vi "localise.vi"() -> ()   [LabVIEW 2016]
panel:
  out "stuff":cluster{dbl, dbl}[](graph)
  out "lidarPos":cluster{"xPos":dbl, "yPos":dbl, "theta":dbl}
  in  "landmarks":cluster{dbl, dbl}[](array[cluster])=[{0.0, 0.0}, {1045.0, 0.0}, {0.0, 4000.0}, {1045.0, 4000.0}, {6000.0, 0.0}, {6000.0, 4000.0}, {5035.0, 0.0}, {5035.0, 4000.0}]
  in  "point merge threshold":dbl=100.0
  out "rotated coordinate system":cluster{"Line":cluster{"X":dbl, "Y":dbl}[]}[](graph)=[{"Line"=[{"X"=4875.364468554468, "Y"=-181.33963012770346}, {"X"=4852.752184853944, "Y"=-189.0958192141975}, {"X"=4830.092735741714, "Y"=-196.71311592818483}, {"X"=4808.9364956042, "Y"=-208.94507233475179}, {"X"=4780.682915441052, "Y"=-199.14542201109134}, {"X"=4754.384597378405, "Y"=-194.86633064519674}, {"X"=4731.399241590487, "Y"=-200.92363554403482}, {"X"=4708.6695027964715, "Y"=-207.79610194101997}, {"X"=4684.775648004498, "Y"=-210.68966547950777}, {"X"=4661.986863653288, "Y"=-217.27587104156783}, {"X"=4639.158096096904, "Y"=-223.7221232680963}, {"X"=4619.181873799431, "Y"=-240.64129637134283}, {"X"=4596.72445242172, "Y"=-248.75730955534345}, {"X"=4573.703746936471, "Y"=-254.80252652544686}, {"X"=4550.156231819835, "Y"=-258.7673691163609}, {"X"=4528.509712831836, "Y"=-270.35259799092773}, {"X"=4496.497729685015, "Y"=-239.02618614387575}, {"X"=4473.538619990259, "Y"=-244.45660669015024}, {"X"=4453.201123871557, "Y"=-261.44876905485853}, {"X"=4430.1052468408925, "Y"=-266.613104523376}, {"X"=4406.978116816861, "Y"=-271.63562913740543}, {"X"=4402.516869914619, "Y"=-366.5963939235294}, {"X"=4378.776773303381, "Y"=-371.44775728191553}, {"X"=4016.6643720573857, "Y"=-184.5155449608328}, {"X"=3994.0487660964363, "Y"=-187.00278952130384}, {"X"=3971.217990913842, "Y"=-187.36127918351485}, {"X"=3948.585779371239, "Y"=-189.56961642142505}, {"X"=3925.5006968150883, "Y"=-186.65841872730198}, {"X"=3902.7918229304946, "Y"=-187.58960731348543}, {"X"=3880.159498496102, "Y"=-189.37808517945405}, {"X"=3857.09903168594, "Y"=-185.04220978622607}, {"X"=3833.975383762099, "Y"=-178.56650338054624}, {"X"=3811.8585360398097, "Y"=-187.9197334957098}, {"X"=3789.2258977826705, "Y"=-189.1502489880163}, {"X"=3766.4959424591943, "Y"=-188.243904779702}, {"X"=3743.862169062455, "Y"=-189.1960745279789}, {"X"=3721.354315175296, "Y"=-194.00719140993715}, {"X"=3698.6593279296276, "Y"=-193.6826253770737}, {"X"=3675.9934601757614, "Y"=-194.2184551012292}, {"X"=3653.324731311072, "Y"=-194.6151995885307}, {"X"=3630.6539948003874, "Y"=-194.8728439017732}, {"X"=3607.97562345001, "Y"=-191.99138534078702}, {"X"=3585.3377427102, "Y"=-187.97085376378345}, {"X"=3562.66860926447, "Y"=-191.81125834809563}, {"X"=3539.951796756734, "Y"=-195.51217198472432}, {"X"=3517.277690740343, "Y"=-195.07415616395292}, {"X"=3494.606699172145, "Y"=-194.4970228896659}, {"X"=3471.939675602154, "Y"=-193.78079389060622}, {"X"=3449.2774734309933, "Y"=-192.92549613238907}, {"X"=3426.6209458777726, "Y"=-191.9311618164934}, {"X"=3403.9709459479454, "Y"=-190.79782837904213}, {"X"=3381.2099975735023, "Y"=-191.52203499291227}, {"X"=3358.3022091020475, "Y"=-194.10153865253824}, {"X"=3335.4973580701767, "Y"=-194.54386256438193}, {"X"=3312.833042285723, "Y"=-192.8513561199734}, {"X"=3289.6776691762902, "Y"=-196.99878969308566}, {"X"=3266.9093951440886, "Y"=-196.02105634650388}, {"X"=3244.141439548919, "Y"=-194.90306841108986}, {"X"=3220.864802139731, "Y"=-198.61872889643155}, {"X"=3197.9614916352934, "Y"=-198.2110591192445}, {"X"=3175.277263429615, "Y"=-195.67457942933152}, {"X"=3152.007693840337, "Y"=-197.9626679594462}, {"X"=3129.3258548014196, "Y"=-195.14422574296668}, {"X"=3106.131977168781, "Y"=-196.1514276372368}, {"X"=3083.462115288954, "Y"=-193.05153141114988}, {"X"=3059.944141155934, "Y"=-195.7495409359385}, {"X"=3036.8256288278494, "Y"=-195.33200506461299}, {"X"=3013.535199662807, "Y"=-195.75743765272819}, {"X"=2989.730023886306, "Y"=-198.99602003762493}, {"X"=2964.5124034139135, "Y"=-209.96651124848268}, {"X"=2941.0609290320317, "Y"=-209.9357542620428}, {"X"=2904.379085672099, "Y"=-281.55213418374296}, {"X"=2789.552062093127, "Y"=-254.5246223646609}, {"X"=2766.529988551289, "Y"=-249.48112943853675}, {"X"=2741.532487512247, "Y"=-253.06988077801316}, {"X"=2718.520244051897, "Y"=-247.73177266645735}, {"X"=2695.5411878061436, "Y"=-242.2525645718888}, {"X"=2669.705574626602, "Y"=-248.2791094206391}, {"X"=2639.072200722142, "Y"=-272.54115478877384}, {"X"=2620.239607261427, "Y"=-250.12607425680517}, {"X"=2600.8696222588273, "Y"=-230.52040448444404}, {"X"=2574.293565720559, "Y"=-237.82052949011359}, {"X"=2551.3780387461265, "Y"=-231.45654971032445}, {"X"=2530.1606574432267, "Y"=-219.18590300588312}, {"X"=2508.4896445348645, "Y"=-208.7142170720531}, {"X"=2484.6010821776836, "Y"=-205.77728069575278}, {"X"=2461.8838573172898, "Y"=-198.86356138814972}, {"X"=2433.210564480137, "Y"=-210.88970641263268}, {"X"=2406.793414706115, "Y"=-215.08573855453687}, {"X"=2384.0205389293933, "Y"=-207.69442514542152}, {"X"=2361.2934440921063, "Y"=-200.16351913679637}, {"X"=2338.6129858565264, "Y"=-192.49330406301624}, {"X"=2315.980018129093, "Y"=-184.68406870334502}, {"X"=2293.395393028246, "Y"=-176.73610707107855}, {"X"=2264.0473517331984, "Y"=-187.45366365313384}, {"X"=2229.322955837718, "Y"=-212.0201293374671}, {"X"=2203.7550913262485, "Y"=-211.02750663514053}, {"X"=2181.0109385315222, "Y"=-202.39044988947717}, {"X"=2158.320209872944, "Y"=-193.61400023597616}, {"X"=2127.189617517972, "Y"=-206.0725272521504}, {"X"=2102.977286469537, "Y"=-200.67385690415676}, {"X"=2078.0144391875347, "Y"=-196.96685847714434}, {"X"=2044.5410314875958, "Y"=-213.38435894728354}, {"X"=2021.785414478626, "Y"=-203.77033872884704}, {"X"=1999.0892163567944, "Y"=-194.01687365053795}]}, {"Line"=[{"X"=995.1561569265573, "Y"=-120.2746516255329}, {"X"=990.8479691186076, "Y"=1267.3599305424295}, {"X"=977.1978637389684, "Y"=1283.4114152543848}, {"X"=963.646505377344, "Y"=1299.5463532737358}, {"X"=944.7929368001387, "Y"=1311.3117052596172}, {"X"=936.8420667751011, "Y"=1332.0641562303358}, {"X"=940.7364779704103, "Y"=1362.2297783899276}, {"X"=992.6762955394938, "Y"=1430.1922552666047}, {"X"=984.7473693279912, "Y"=1449.9310553634696}, {"X"=983.2886202921791, "Y"=1474.5858311674642}, {"X"=1038.4449660668279, "Y"=1542.2942488382926}, {"X"=1026.4809299503295, "Y"=1558.048508306483}, {"X"=1014.6137853722585, "Y"=1573.875881150741}, {"X"=976.2601861062503, "Y"=1570.223228197419}, {"X"=957.9951708726335, "Y"=1581.6581423355021}, {"X"=946.2741815106342, "Y"=1597.9052914528809}, {"X"=941.18381557668, "Y"=1618.8446376100087}, {"X"=1035.4542316465918, "Y"=1709.0536015780297}, {"X"=1037.6873121359445, "Y"=1733.9032615366507}, {"X"=1035.1673005512534, "Y"=1755.2830533755748}, {"X"=1032.8128759176288, "Y"=1776.627065912406}, {"X"=1034.7918620045143, "Y"=1800.6953749366378}, {"X"=1024.4134141596182, "Y"=1816.4671851017908}, {"X"=1015.8127079164447, "Y"=1833.3863556799192}, {"X"=1025.8839062712937, "Y"=1862.1577194348454}, {"X"=1020.9645951345497, "Y"=1881.1728379933504}, {"X"=1006.82910819158, "Y"=1894.3958377366096}, {"X"=1030.3100502453976, "Y"=1930.6642927244054}, {"X"=1030.1519372868106, "Y"=1952.136655072785}, {"X"=1029.3004603365107, "Y"=1973.040970826681}, {"X"=1034.6486208208826, "Y"=1997.4350924689477}, {"X"=1036.7349309586402, "Y"=2019.7053719504383}, {"X"=1052.0328316602431, "Y"=2049.314882869931}, {"X"=1044.923639308267, "Y"=2065.955094484733}, {"X"=1052.7981056635122, "Y"=2090.857172076369}, {"X"=1044.1997181730085, "Y"=2106.513035793635}, {"X"=1035.697555118571, "Y"=2122.2213635075027}, {"X"=1027.2919366018336, "Y"=2137.9815638083105}, {"X"=973.7644027699575, "Y"=2130.2078304203374}, {"X"=1038.1094935815977, "Y"=2647.5230014110284}, {"X"=1052.8931430954117, "Y"=2669.7665030188023}, {"X"=1057.3733887850622, "Y"=2688.4515319824445}, {"X"=1052.4416852255154, "Y"=2704.0680727452964}, {"X"=1047.6058957966343, "Y"=2719.714579895345}, {"X"=1053.4051578916715, "Y"=2738.5417213351366}, {"X"=1051.6603564800585, "Y"=2755.023449184703}, {"X"=1050.021828763001, "Y"=2771.4978886682547}, {"X"=1046.5630241118151, "Y"=2787.4267685584864}, {"X"=1045.133311119083, "Y"=2803.8964142840096}, {"X"=1046.7087363121373, "Y"=2821.12760935855}, {"X"=1054.2071036963334, "Y"=2839.819320844825}, {"X"=1053.1127473126949, "Y"=2856.1876654653834}, {"X"=1056.978250286315, "Y"=2873.7401653601373}, {"X"=1053.1834638463438, "Y"=2889.3556426410773}, {"X"=1061.1707740855086, "Y"=2907.720368708814}, {"X"=1058.5596338716723, "Y"=2923.5306899638895}, {"X"=1080.4610293828596, "Y"=2944.731258270807}, {"X"=1079.05712939688, "Y"=2960.6197601364106}, {"X"=1075.7950105001619, "Y"=2976.0981284781265}, {"X"=1075.5690111418248, "Y"=2992.187847238236}, {"X"=1072.5006560489983, "Y"=3007.6870240108883}, {"X"=1057.7349664870621, "Y"=3020.982777577399}, {"X"=1016.4744379708436, "Y"=3029.6047721947734}, {"X"=985.074506559165, "Y"=3040.446234099636}, {"X"=961.5990224884686, "Y"=3052.991854810011}, {"X"=958.9058992251366, "Y"=3069.189193668247}, {"X"=932.602007282233, "Y"=3081.6843913440134}, {"X"=1024.2156184414202, "Y"=3176.6568081451514}, {"X"=1032.2096938775303, "Y"=3193.652250239258}, {"X"=1030.378317349322, "Y"=3209.413682270658}, {"X"=1028.6436856251103, "Y"=3225.1860547126794}, {"X"=1024.0209520220938, "Y"=3240.668273481939}, {"X"=1022.4782145399163, "Y"=3256.479065625435}]}, {"Line"=[{"X"=-27.88704701562665, "Y"=3179.6883172654543}, {"X"=-29.784148604247548, "Y"=3201.9546434830118}, {"X"=-40.51875378113118, "Y"=3223.5507218893886}, {"X"=-42.14648292623542, "Y"=3245.8937291052093}, {"X"=-43.63708731480574, "Y"=3268.2463032785063}, {"X"=-42.9938027953026, "Y"=3290.7223069817924}, {"X"=-44.20932825047976, "Y"=3313.079236326757}, {"X"=-45.287651284163985, "Y"=3335.4432031328274}, {"X"=-45.22949075787301, "Y"=3357.852331327238}, {"X"=-44.03415040060372, "Y"=3380.287382811384}, {"X"=-44.70009529764866, "Y"=3402.64900957201}, {"X"=-45.22881929609821, "Y"=3425.0143015424014}, {"X"=-45.620302489793175, "Y"=3447.3824166819586}, {"X"=-45.874530139612034, "Y"=3469.7525128437887}, {"X"=-45.99149267402754, "Y"=3492.1237478064127}, {"X"=-45.97118568946689, "Y"=3514.49527930548}, {"X"=-44.81366107226677, "Y"=3536.8561536378656}, {"X"=-45.518771389693484, "Y"=3559.235862831427}, {"X"=-44.086931606495455, "Y"=3581.580848823444}, {"X"=-43.51776202187057, "Y"=3603.939010150847}, {"X"=-42.81141605282983, "Y"=3626.293258233267}, {"X"=-42.967088446615435, "Y"=3648.6835313502697}, {"X"=-45.98180211856061, "Y"=3671.2211979291474}, {"X"=-48.856943965644405, "Y"=3693.801451165101}, {"X"=-47.59911191565743, "Y"=3716.1867682169914}, {"X"=-46.20394982073867, "Y"=3738.563945959246}, {"X"=-44.67151020795109, "Y"=3760.9321419037724}, {"X"=-51.97476173527639, "Y"=3783.988273787092}, {"X"=-52.15648631405884, "Y"=3806.558313333936}, {"X"=-50.206729051451475, "Y"=3828.9617533810065}, {"X"=-46.12875527743017, "Y"=3851.161074065816}, {"X"=-43.90543409027123, "Y"=3873.5266890161834}]}, {"Line"=[{"X"=-57.451206048306176, "Y"=3897.6074387832673}, {"X"=1335.6105985632566, "Y"=3873.584848007716}, {"X"=1337.9454985878674, "Y"=3887.471847546513}, {"X"=1353.1652358742085, "Y"=3899.0708492433396}, {"X"=1355.6561846014824, "Y"=3912.8496557857657}, {"X"=1820.0951553792638, "Y"=3850.049630903437}, {"X"=1822.2765257416634, "Y"=3860.964332131124}, {"X"=1949.8064262901478, "Y"=3845.6257647900497}, {"X"=2047.7518614123712, "Y"=3835.0667340265845}, {"X"=2074.2413420170706, "Y"=3839.160017676214}, {"X"=2132.890864786777, "Y"=3835.582754881576}, {"X"=2166.127558146054, "Y"=3837.251865067938}, {"X"=2200.3003394848, "Y"=3838.2910881971834}, {"X"=2248.018436192918, "Y"=3835.5515625440557}, {"X"=2277.236404755542, "Y"=3836.9294749587143}, {"X"=2307.3868846214937, "Y"=3837.7089485806855}, {"X"=2344.25776130767, "Y"=3836.3204275151534}, {"X"=2371.41812317585, "Y"=3837.1388021857606}, {"X"=2396.6148897993025, "Y"=3838.177877081358}, {"X"=2414.0890428141442, "Y"=3841.132234810093}, {"X"=2450.739877896451, "Y"=3838.2383357080275}, {"X"=2474.8609031479305, "Y"=3838.6547101915307}, {"X"=2494.1640463756876, "Y"=3840.2584953705154}, {"X"=2511.535949867143, "Y"=3842.238238027806}, {"X"=2537.4588200341204, "Y"=3841.26564561455}, {"X"=2560.4772677834208, "Y"=3840.9229960049315}, {"X"=2579.6576251688384, "Y"=3841.5807929669136}, {"X"=2592.1821197265217, "Y"=3844.2791312308555}, {"X"=2624.5313575165155, "Y"=3839.926356041171}, {"X"=2642.654053105019, "Y"=3840.2127833632244}, {"X"=2653.221356629601, "Y"=3843.014869149585}, {"X"=2670.353311050435, "Y"=3843.2754487654347}, {"X"=2686.5163060590426, "Y"=3843.6910544427697}, {"X"=2712.9203209596462, "Y"=3839.9847688259915}, {"X"=2718.749345719235, "Y"=3843.9669814527606}, {"X"=2735.745373534478, "Y"=3843.4587902979656}, {"X"=2759.190584115213, "Y"=3840.130160614261}, {"X"=2762.2181156127335, "Y"=3844.902180614331}, {"X"=2778.185428757569, "Y"=3844.2409192609425}, {"X"=2791.3526756724646, "Y"=3844.5729311160676}, {"X"=2798.98739923077, "Y"=3847.1423532341078}, {"X"=2804.792835674701, "Y"=3850.437677491615}, {"X"=2817.9091475083846, "Y"=3850.4039075822907}, {"X"=2837.3651516827986, "Y"=3847.321303884745}, {"X"=2852.215704506808, "Y"=3846.113633672166}, {"X"=2861.5927811261063, "Y"=3847.2906262986685}, {"X"=2874.5650046463807, "Y"=3846.6411220791524}, {"X"=2883.9025697924535, "Y"=3847.5923912431745}, {"X"=2896.8119198019726, "Y"=3846.6735119206733}, {"X"=2900.740692773926, "Y"=3850.0863054415463}, {"X"=2910.9248129571906, "Y"=3850.291859171631}, {"X"=2923.750724150955, "Y"=3849.0099094777147}, {"X"=2930.33394718425, "Y"=3850.832406864265}, {"X"=2937.7968458711803, "Y"=3852.1178533699235}, {"X"=2955.810589401053, "Y"=3847.6262407704303}, {"X"=2966.7268074487856, "Y"=3846.769467508303}, {"X"=2977.607927778653, "Y"=3845.7920016946864}, {"X"=2984.9682824182264, "Y"=3846.658313571755}, {"X"=2988.8431566734257, "Y"=3849.432844556857}, {"X"=3000.514385824566, "Y"=3847.6578754993225}, {"X"=3004.3827878484135, "Y"=3850.315766971416}, {"X"=3013.414194881955, "Y"=3849.8658217574493}, {"X"=3017.2833293798044, "Y"=3852.4234410213294}, {"X"=3034.8014845147404, "Y"=3846.582801208108}, {"X"=3037.787979177994, "Y"=3849.5162995387154}, {"X"=3053.4792714726036, "Y"=3844.4286476033662}, {"X"=3057.2883738551773, "Y"=3846.698847484733}, {"X"=3063.622898309917, "Y"=3847.304772185103}, {"X"=3067.436117579296, "Y"=3849.492075934472}, {"X"=3070.4232538474694, "Y"=3852.199474636885}, {"X"=3088.3501096376754, "Y"=3844.823708135362}, {"X"=3090.4755397996805, "Y"=3847.956641634519}, {"X"=3092.620153269628, "Y"=3851.0764747627854}, {"X"=3108.7039247689136, "Y"=3844.4243987619507}, {"X"=3110.8265216598475, "Y"=3847.432451116179}, {"X"=3113.779256429665, "Y"=3849.8433771302675}, {"X"=3119.167495430773, "Y"=3850.46412448307}, {"X"=3125.3494169762807, "Y"=3850.4380459300096}, {"X"=3131.5127639763296, "Y"=3850.3494108499426}, {"X"=3136.859859086742, "Y"=3850.8022375567853}, {"X"=3141.401329549159, "Y"=3851.811397570802}, {"X"=3149.8860258047935, "Y"=3849.7104662920415}, {"X"=3156.755647605926, "Y"=3848.755564931598}, {"X"=3160.4680859852774, "Y"=3850.2223530309775}, {"X"=3169.629505439559, "Y"=3847.2610508130756}, {"X"=3172.5427398878355, "Y"=3849.262495520778}, {"X"=3178.5462320761003, "Y"=3848.691441682683}, {"X"=3183.7599215441505, "Y"=3848.7021610014317}, {"X"=3186.6699549419614, "Y"=3850.602729385154}, {"X"=3191.1048479470255, "Y"=3851.1776681789074}, {"X"=3199.3041794662954, "Y"=3848.4305661201684}, {"X"=3205.953045974128, "Y"=3846.91785486327}, {"X"=3208.0891117368533, "Y"=3849.3291508889447}, {"X"=3211.7247329793054, "Y"=3850.3873813652654}, {"X"=3220.5264570839636, "Y"=3846.6927028749683}, {"X"=3224.129112653411, "Y"=3847.656548975117}, {"X"=3226.2693687986784, "Y"=3849.9563048465648}, {"X"=3229.875165629684, "Y"=3850.866936291162}, {"X"=3232.7565121495086, "Y"=3852.4389601497064}, {"X"=3239.9466149416203, "Y"=3849.8078900025016}, {"X"=3245.66451699703, "Y"=3848.504469820765}, {"X"=3249.935468453753, "Y"=3848.5553381506397}, {"X"=3254.193623585364, "Y"=3848.566995039661}, {"X"=3257.0388209403313, "Y"=3849.9680409094553}, {"X"=3266.843418073042, "Y"=3844.1623046162176}, {"X"=3268.961429853259, "Y"=3846.2000362149047}, {"X"=3273.1518722403007, "Y"=3846.0437853508993}, {"X"=3275.281309814408, "Y"=3848.0427735841577}, {"X"=3278.1006556937873, "Y"=3849.2933038797487}, {"X"=3283.6157288974155, "Y"=3847.564372453343}, {"X"=3287.091515385653, "Y"=3848.0118967166973}, {"X"=3293.2169619535393, "Y"=3845.43909386024}, {"X"=3297.98004039561, "Y"=3844.307920327957}, {"X"=3298.1339382930623, "Y"=3848.4219866620697}, {"X"=3302.227969769491, "Y"=3847.9882440721253}, {"X"=3304.368790968698, "Y"=3849.8087881210113}, {"X"=3309.0838801357822, "Y"=3848.5452785552375}, {"X"=3315.044360347663, "Y"=3845.6939158132923}, {"X"=3317.1708625483957, "Y"=3847.4358631580535}, {"X"=3319.9345577199, "Y"=3848.3853441814854}, {"X"=3322.077482158057, "Y"=3850.09723517388}, {"X"=3324.2308702219293, "Y"=3851.7959452032464}, {"X"=3327.006733363762, "Y"=3852.6906241612837}, {"X"=3334.033772019595, "Y"=3848.002824088936}, {"X"=3337.3787684930608, "Y"=3848.03173527967}, {"X"=3339.5191948454476, "Y"=3849.6365972635535}, {"X"=3341.6694281529244, "Y"=3851.2282956271647}, {"X"=3346.767123842757, "Y"=3848.7608212416217}, {"X"=3348.9118470493695, "Y"=3850.3080636351965}, {"X"=3352.7987426764153, "Y"=3849.393100071594}, {"X"=3354.9472319294746, "Y"=3850.9033212452873}, {"X"=3358.239970891585, "Y"=3850.7536005880743}, {"X"=3360.959154637208, "Y"=3851.403577455099}, {"X"=3363.677191444651, "Y"=3852.0334219310885}, {"X"=3365.2894164277122, "Y"=3854.310516297719}, {"X"=3371.844919137942, "Y"=3849.0476458548715}, {"X"=3373.9909301848866, "Y"=3850.4410083898674}, {"X"=3376.145450345569, "Y"=3851.821177018968}, {"X"=3379.371667575448, "Y"=3851.4941520588377}, {"X"=3384.69111397845, "Y"=3847.7399654916867}, {"X"=3386.828859423541, "Y"=3849.054529873674}, {"X"=3390.0065395382076, "Y"=3848.6427205080895}, {"X"=3392.6604127610813, "Y"=3849.064887325544}, {"X"=3394.300734152325, "Y"=3851.193411142247}, {"X"=3398.459886789198, "Y"=3848.9850752782663}, {"X"=3401.5945661769583, "Y"=3848.4770922592916}, {"X"=3402.7576461014837, "Y"=3851.4320045593067}, {"X"=3405.885855720585, "Y"=3850.8855924523987}, {"X"=3410.4359883800344, "Y"=3847.6801482663996}, {"X"=3412.5728821535454, "Y"=3848.836746194794}, {"X"=3413.781058878635, "Y"=3851.7477874381552}, {"X"=3416.8677585572095, "Y"=3851.1104984818016}, {"X"=3419.0255794876925, "Y"=3852.227567234926}, {"X"=3422.5448335937085, "Y"=3850.6546219796846}, {"X"=3424.699750449227, "Y"=3851.7368654369866}, {"X"=3426.8612672600616, "Y"=3852.805866200107}, {"X"=3429.8993825310763, "Y"=3852.060761711229}, {"X"=3432.921802718256, "Y"=3851.2917249140414}, {"X"=3437.200222193895, "Y"=3847.781874666123}, {"X"=3439.337236319723, "Y"=3848.7742484281425}, {"X"=3442.3059227489016, "Y"=3847.9318582710193}, {"X"=3444.8509763286847, "Y"=3847.979569017834}, {"X"=3446.5874559424906, "Y"=3849.8408085484066}, {"X"=3448.736926737098, "Y"=3850.7755445681214}, {"X"=3450.8920925009197, "Y"=3851.6970740868423}, {"X"=3451.129480366653, "Y"=3857.220615844183}, {"X"=3453.324147305234, "Y"=3858.1273436031706}, {"X"=3456.6443028904364, "Y"=3856.237482736209}, {"X"=3459.935702110019, "Y"=3854.320465760287}, {"X"=3462.1124082875845, "Y"=3855.173214152968}, {"X"=3466.787586324898, "Y"=3849.471676739122}, {"X"=3469.2848546564674, "Y"=3849.3458898825334}, {"X"=3471.4308614151137, "Y"=3850.1413665986074}, {"X"=3473.920631762058, "Y"=3849.982846586403}, {"X"=3476.7367473982727, "Y"=3848.8641147467633}, {"X"=3478.8796577604844, "Y"=3849.6138765778364}, {"X"=3481.670224839258, "Y"=3848.4566892892262}, {"X"=3483.81054241454, "Y"=3849.1761875414713}, {"X"=3485.3354259488456, "Y"=3851.784075048413}, {"X"=3487.192026363989, "Y"=3853.4336728215594}, {"X"=3489.362778189773, "Y"=3854.1191962462844}, {"X"=3491.537695444426, "Y"=3854.79138728342}, {"X"=3493.716696243542, "Y"=3855.4502206253537}, {"X"=3497.0220737667746, "Y"=3852.2563650364664}, {"X"=3500.009514130937, "Y"=3849.9970038952742}, {"X"=3502.6965259216036, "Y"=3848.677550083562}, {"X"=3504.837802859068, "Y"=3849.2680292201253}, {"X"=3506.9826625994683, "Y"=3849.8453586127957}, {"X"=3508.6289858507666, "Y"=3852.345480705146}, {"X"=3510.7926571105445, "Y"=3852.8994899041413}, {"X"=3512.9596869763614, "Y"=3853.4402126368004}, {"X"=3515.1299938607685, "Y"=3853.96762854522}, {"X"=3517.3034960529376, "Y"=3854.481717772487}, {"X"=3520.1437371745833, "Y"=3852.05678134011}, {"X"=3522.7358611314803, "Y"=3850.5870118029275}, {"X"=3525.5161499645315, "Y"=3848.120892914938}, {"X"=3527.4503614688483, "Y"=3849.550496994353}, {"X"=3529.596528723903, "Y"=3849.9890730183956}, {"X"=3531.7453466298593, "Y"=3850.4144721516536}, {"X"=3533.896734284937, "Y"=3850.82667837809}, {"X"=3536.050610690607, "Y"=3851.2256761783733}, {"X"=3538.2068947546404, "Y"=3851.6114505304627}, {"X"=3540.6995920992354, "Y"=3850.012087823839}, {"X"=3543.0093327946784, "Y"=3849.3824034657328}, {"X"=3545.154175753993, "Y"=3849.7255146007737}, {"X"=3547.301083627591, "Y"=3850.0554587678553}, {"X"=3549.449975585606, "Y"=3850.3722235447667}, {"X"=3551.737491710125, "Y"=3849.6851874094323}, {"X"=3553.8840282116666, "Y"=3849.9747378683464}, {"X"=3556.156855341715, "Y"=3849.258899194384}, {"X"=3558.1822290543146, "Y"=3850.5142993276227}, {"X"=3560.446100602967, "Y"=3849.7706234698526}, {"X"=3562.5929973932184, "Y"=3850.006737300836}, {"X"=3564.7413025359765, "Y"=3850.229673575984}, {"X"=3566.890935148765, "Y"=3850.439423901873}, {"X"=3569.0418142991325, "Y"=3850.635980381521}, {"X"=3571.0301877520556, "Y"=3852.8126272943173}, {"X"=3573.195550684427, "Y"=3852.9837411225744}, {"X"=3575.361922789166, "Y"=3853.141565312486}, {"X"=3577.529222503586, "Y"=3853.28609392206}, {"X"=3579.6973682300777, "Y"=3853.417321509876}, {"X"=3581.866278339181, "Y"=3853.535243135289}, {"X"=3584.035871172656, "Y"=3853.639854358617}, {"X"=3586.206065046558, "Y"=3853.7311512413066}, {"X"=3588.376778254314, "Y"=3853.8091303460815}, {"X"=3590.5479290698, "Y"=3853.8737887370726}, {"X"=3592.7194357504145, "Y"=3853.9251239799287}, {"X"=3594.862353356768, "Y"=3855.962925860221}, {"X"=3597.0383014495974, "Y"=3856.9877145528917}, {"X"=3599.2287926403974, "Y"=3856.9991670007207}, {"X"=3601.4193128667184, "Y"=3856.997178631689}, {"X"=3603.650225367152, "Y"=3860.9815450334945}, {"X"=3605.735123307596, "Y"=3852.953408200922}, {"X"=3607.900696744767, "Y"=3852.911573897694}, {"X"=3610.00894171823, "Y"=3850.8572659724764}, {"X"=3612.3001664397284, "Y"=3854.7868457335403}, {"X"=3614.3545263399055, "Y"=3851.707190107846}, {"X"=3616.5592007860246, "Y"=3852.611390725439}, {"X"=3618.7224718832185, "Y"=3852.5031475697515}, {"X"=3620.885038089928, "Y"=3852.381632869794}, {"X"=3623.046817986758, "Y"=3852.2468512005257}, {"X"=3625.2077301839167, "Y"=3852.0988076364006}, {"X"=3627.290164448009, "Y"=3850.940517644231}, {"X"=3629.2756915871423, "Y"=3848.7734707257623}, {"X"=3631.594689547098, "Y"=3850.579200170835}, {"X"=3633.265872973202, "Y"=3845.401768517955}, {"X"=3635.3845921617844, "Y"=3845.1911508679564}, {"X"=3637.7181288761512, "Y"=3846.955822481886}, {"X"=3640.0746453054317, "Y"=3848.704778865509}, {"X"=3642.2135032112865, "Y"=3848.452321195642}, {"X"=3644.3507718026044, "Y"=3848.186744492827}, {"X"=3646.8836900193755, "Y"=3850.8816319076377}, {"X"=3649.451334095426, "Y"=3853.558433015227}, {"X"=3651.1860171434532, "Y"=3850.2798761690287}, {"X"=3653.334330496239, "Y"=3849.9592107525073}, {"X"=3655.4806358416267, "Y"=3849.625369569499}, {"X"=3657.4620703035835, "Y"=3848.2917031403795}, {"X"=3659.260400212996, "Y"=3845.961276686561}, {"X"=3661.3820631395324, "Y"=3845.5911490833273}, {"X"=3663.863246490962, "Y"=3847.175007377597}, {"X"=3666.7400578446986, "Y"=3850.7060944421787}, {"X"=3668.8906936232233, "Y"=3850.289983202648}, {"X"=3671.0387357060704, "Y"=3849.860683743234}, {"X"=3673.1841032206685, "Y"=3849.4182122268194}, {"X"=3675.537714597933, "Y"=3849.9400715455736}, {"X"=3677.683484534923, "Y"=3849.469993319187}, {"X"=3679.8263297326275, "Y"=3848.9867577450727}, {"X"=3681.9661695141353, "Y"=3848.4903830167773}, {"X"=3684.572772049296, "Y"=3849.9249151288}, {"X"=3686.95916301393, "Y"=3850.3699530038452}, {"X"=3688.8605208682325, "Y"=3848.8607284161208}, {"X"=3691.2521934413376, "Y"=3849.2764480925457}, {"X"=3693.3935956407463, "Y"=3848.7099601291775}, {"X"=3696.3253720530747, "Y"=3851.0233933783284}, {"X"=3698.4773978060916, "Y"=3850.425744090443}, {"X"=3700.6257159407405, "Y"=3849.8149014713545}, {"X"=3702.2055738950803, "Y"=3847.272257263343}, {"X"=3703.758038867192, "Y"=3844.7234679716976}, {"X"=3705.8712690867633, "Y"=3844.0803312919206}, {"X"=3708.5804050535194, "Y"=3845.332152627602}]}]
  out "angle deviation":dbl=-12.54564800056658 format="%0.2f"
  in  "max angle deviation":dbl=30.0
  out "split&merge":cluster{"Line":cluster{"X":dbl, "Y":dbl}[]}[](graph)=[{"Line"=[{"X"=4045.262015510834, "Y"=-370.47254705975547}, {"X"=4021.5048604927456, "Y"=-373.1317628736815}, {"X"=3997.731836054895, "Y"=-375.64515746583857}, {"X"=3974.4237446268694, "Y"=-382.9895518092235}, {"X"=3948.973422153729, "Y"=-367.28671688954455}, {"X"=3924.2325152064327, "Y"=-357.3973448535103}, {"X"=3900.4802229985116, "Y"=-358.3172025621179}, {"X"=3876.8003772484603, "Y"=-360.08828281881506}, {"X"=3852.848497603733, "Y"=-357.72259724044125}, {"X"=3829.173196937117, "Y"=-359.2014259177531}, {"X"=3805.4892680291655, "Y"=-360.5349578426094}, {"X"=3782.314874586134, "Y"=-372.7109737888577}, {"X"=3758.6307242397825, "Y"=-375.7550610593494}, {"X"=3734.846552078191, "Y"=-376.65544089136483}, {"X"=3711.0000422297094, "Y"=-375.4106867047012}, {"X"=3687.3538586650116, "Y"=-382.0172981809769}, {"X"=3662.9108581038413, "Y"=-344.48530026226535}, {"X"=3639.320355486937, "Y"=-344.7989426814479}, {"X"=3615.7774597291873, "Y"=-356.96773019486045}, {"X"=3592.111253634981, "Y"=-356.9919325402784}, {"X"=3568.4453445476156, "Y"=-356.8709213194161}, {"X"=3543.4634903042615, "Y"=-448.5952721279782}, {"X"=3519.2364294721056, "Y"=-448.174039435899}, {"X"=3206.375015694224, "Y"=-187.04805660711145}, {"X"=3183.7591240020847, "Y"=-184.5634114706845}, {"X"=3161.3956031641924, "Y"=-179.95410067521016}, {"X"=3138.8240858920867, "Y"=-177.1936005936277}, {"X"=3116.9225625935896, "Y"=-169.33743194447243}, {"X"=3094.5536322950015, "Y"=-165.31362496769452}, {"X"=3072.0732055742583, "Y"=-162.14326586595462}, {"X"=3050.50517501786, "Y"=-152.90178314690638}, {"X"=3029.3402803672284, "Y"=-141.5578375729042}, {"X"=3005.7198268817183, "Y"=-145.8835795782761}, {"X"=2983.360292949494, "Y"=-142.16851225868822}, {"X"=2961.369928605174, "Y"=-136.34646752894514}, {"X"=2939.069748166673, "Y"=-132.35945388277014}, {"X"=2916.0542503508345, "Y"=-132.16660019014535}, {"X"=2893.971646836575, "Y"=-126.92003834235948}, {"X"=2871.7305746338234, "Y"=-122.51965406356612}, {"X"=2849.516921363317, "Y"=-117.98288396725366}, {"X"=2827.3315233565468, "Y"=-113.3098988602519}, {"X"=2805.820540469126, "Y"=-105.57110400824695}, {"X"=2784.596507850818, "Y"=-96.72922875644326}, {"X"=2761.6344368770942, "Y"=-95.5538074919159}, {"X"=2738.656125118518, "Y"=-94.23186914869939}, {"X"=2716.6185475221346, "Y"=-88.87910208996846}, {"X"=2694.614228738148, "Y"=-83.39121576148591}, {"X"=2672.6439972167227, "Y"=-77.76841677907123}, {"X"=2650.708680124659, "Y"=-72.01091683792765}, {"X"=2628.809103314247, "Y"=-66.11893270467408}, {"X"=2606.946091292176, "Y"=-60.092686209182375}, {"X"=2584.5712899521213, "Y"=-55.85552783159346}, {"X"=2561.650151837172, "Y"=-53.3974718317445}, {"X"=2539.293725910705, "Y"=-48.87562477295114}, {"X"=2517.538201938755, "Y"=-42.30044684778477}, {"X"=2494.034809091436, "Y"=-41.3191040202214}, {"X"=2472.0225479250194, "Y"=-35.41905120318597}, {"X"=2450.0410633250167, "Y"=-29.382161789984366}, {"X"=2426.5130901879893, "Y"=-27.95301449719682}, {"X"=2404.2451890722396, "Y"=-22.58008172179325}, {"X"=2382.6535537697796, "Y"=-15.176756558716079}, {"X"=2359.4425731187703, "Y"=-12.355658331004179}, {"X"=2337.9145170954243, "Y"=-4.677621956337134}, {"X"=2315.0556519473794, "Y"=-0.6226620999336774}, {"X"=2293.6004238067435, "Y"=7.327506432634436}, {"X"=2270.057927743648, "Y"=9.802429024614412}, {"X"=2247.5821062096375, "Y"=15.231737897677704}, {"X"=2224.75536526262, "Y"=19.875548974426238}, {"X"=2200.815103181707, "Y"=21.88519100999474}, {"X"=2173.8166160981887, "Y"=16.65434452990621}, {"X"=2150.9317674680565, "Y"=21.778434678614303}, {"X"=2099.569445467065, "Y"=-40.16004596176299}, {"X"=1993.354962067471, "Y"=11.164560761459143}, {"X"=1971.9781148912214, "Y"=21.088425727543836}, {"X"=1946.7979336116412, "Y"=23.015253457493145}, {"X"=1925.494677341689, "Y"=33.224563893850245}, {"X"=1904.2544652507022, "Y"=43.564396465946174}, {"X"=1877.726652128255, "Y"=43.29368976613068}, {"X"=1842.55456574985, "Y"=26.26504384210375}, {"X"=1829.0405780564897, "Y"=52.23569166488596}, {"X"=1814.3917771697875, "Y"=75.5807390798177}, {"X"=1786.8645563340388, "Y"=74.22769832520271}, {"X"=1765.8785444190275, "Y"=85.41737745628188}, {"X"=1747.8331626322108, "Y"=102.00382481748511}, {"X"=1728.9542149611082, "Y"=116.9328013933573}, {"X"=1706.27398723018, "Y"=124.98862393636955}, {"X"=1685.60095559409, "Y"=136.67184194320134}, {"X"=1655.000000000001, "Y"=131.16117927853338}, {"X"=1628.3021546343343, "Y"=132.80359845458497}, {"X"=1607.6785425781395, "Y"=144.9650955174202}, {"X"=1587.1299402987506, "Y"=157.25290774813675}, {"X"=1566.6571214394316, "Y"=169.66657251754714}, {"X"=1546.2608567902394, "Y"=182.2056224581911}, {"X"=1525.9419142590123, "Y"=194.86958548192388}, {"X"=1494.9665691389255, "Y"=190.7828335152658}, {"X"=1455.735015665709, "Y"=174.34567686930814}, {"X"=1430.993243345882, "Y"=180.86838320792322}, {"X"=1410.668265549114, "Y"=194.23964018468632}, {"X"=1390.425714854734, "Y"=207.7353571705712}, {"X"=1357.3322111709276, "Y"=202.3364045208432}, {"X"=1334.8706766640394, "Y"=212.86551103190004}, {"X"=1311.3090852839077, "Y"=221.9063623965808}, {"X"=1275.0687472590512, "Y"=213.15186386282812}, {"X"=1254.9447924102292, "Y"=227.47924783415692}, {"X"=1234.9091275645433, "Y"=241.92984036216785}]}, {"Line"=[{"X"=270.96481001367874, "Y"=531.983035117094}, {"X"=568.1778192565093, "Y"=1887.4212377834735}, {"X"=558.3402951796288, "Y"=1906.0545053007447}, {"X"=548.617287871481, "Y"=1924.7477839649912}, {"X"=532.7695198753122, "Y"=1940.3275402206798}, {"X"=529.5162834990319, "Y"=1962.3115573360112}, {"X"=539.8702058904678, "Y"=1990.9109889727677}, {"X"=605.3325001870285, "Y"=2045.968512870534}, {"X"=601.8805011027116, "Y"=2066.9583152148466}, {"X"=605.8120277476805, "Y"=2091.3412809272986}, {"X"=674.3588639641607, "Y"=2145.452125934663}, {"X"=666.1025888247354, "Y"=2163.429021451132}, {"X"=657.9567732645942, "Y"=2181.4562381095116}, {"X"=619.7255133273352, "Y"=2186.221866490394}, {"X"=604.3804690989409, "Y"=2201.3512306693083}, {"X"=596.4685017416655, "Y"=2219.7564532597535}, {"X"=596.0480668191567, "Y"=2241.301551943805}, {"X"=707.6625662145384, "Y"=2308.879448114789}, {"X"=715.2401057472161, "Y"=2332.650715290977}, {"X"=717.4243259383866, "Y"=2354.0674176426273}, {"X"=719.7624075179106, "Y"=2375.413226623674}, {"X"=726.9221966011937, "Y"=2398.476992697342}, {"X"=720.2174633677091, "Y"=2416.1266025463633}, {"X"=715.4972516675775, "Y"=2434.5100212284015}, {"X"=731.5776225251552, "Y"=2460.4067793595614}, {"X"=730.9061825143826, "Y"=2480.0364386578276}, {"X"=719.9804701443845, "Y"=2496.014189517481}, {"X"=750.778902136793, "Y"=2526.316203538756}, {"X"=755.2887344326768, "Y"=2547.3102207148654}, {"X"=758.99836842379, "Y"=2567.9003650996783}, {"X"=769.5176591565032, "Y"=2590.550321252946}, {"X"=776.3916464972967, "Y"=2611.8356762232834}, {"X"=797.7559831999147, "Y"=2637.415238768894}, {"X"=794.4310781670474, "Y"=2655.202376397113}, {"X"=807.5266916718274, "Y"=2677.7994026548567}, {"X"=802.5343311689248, "Y"=2694.949174454491}, {"X"=797.6472936673199, "Y"=2712.1292559626913}, {"X"=792.8657631612118, "Y"=2729.3390003590985}, {"X"=738.9277025317801, "Y"=2733.377988406333}, {"X"=914.1062820436955, "Y"=3224.364487333619}, {"X"=933.3686210466781, "Y"=3242.8656211598604}, {"X"=941.800605877364, "Y"=3260.131325333941}, {"X"=940.3788392110519, "Y"=3276.4462456507435}, {"X"=939.0572057782192, "Y"=3292.769582640043}, {"X"=948.8075824980851, "Y"=3309.887492835553}, {"X"=950.6845588015076, "Y"=3326.35469189397}, {"X"=952.6636881702325, "Y"=3342.7916921165966}, {"X"=952.7474978684022, "Y"=3359.091554695986}, {"X"=954.9294148586805, "Y"=3375.478517435108}, {"X"=960.2101388711521, "Y"=3391.956077999096}, {"X"=971.5896340437512, "Y"=3408.572716688413}, {"X"=974.0768960605492, "Y"=3424.7879517829642}, {"X"=981.6628112449193, "Y"=3441.081700787105}, {"X"=981.3505848148575, "Y"=3457.1486248702304}, {"X"=993.1363215681313, "Y"=3473.3398786074254}, {"X"=994.0218032440225, "Y"=3489.3398859076315}, {"X"=1020.0053964340373, "Y"=3505.2768902312037}, {"X"=1022.0862755609401, "Y"=3521.09097789895}, {"X"=1022.2642158658068, "Y"=3536.908362115882}, {"X"=1025.5385789953302, "Y"=3552.663001800286}, {"X"=1025.91017660836, "Y"=3568.4586087471434}, {"X"=1014.3851121986418, "Y"=3584.6442672599346}, {"X"=975.9825976478487, "Y"=3602.0229001404546}, {"X"=947.6873481122784, "Y"=3619.426113711875}, {"X"=927.497508824365, "Y"=3636.771468735349}, {"X"=928.3870318839645, "Y"=3653.1670610615342}, {"X"=905.4253651296312, "Y"=3671.0775763015645}, {"X"=1015.481200145904, "Y"=3743.8822937417594}, {"X"=1026.9761083045855, "Y"=3758.735488027024}, {"X"=1028.6121158613832, "Y"=3774.518395203543}, {"X"=1030.3449347186652, "Y"=3790.29096691764}, {"X"=1029.195583743087, "Y"=3806.4076587716963}, {"X"=1031.1240604595514, "Y"=3822.1760500878013}]}, {"Line"=[{"X"=-10.842185123417494, "Y"=3975.376392065428}, {"X"=-7.85735733306592, "Y"=3997.523154373408}, {"X"=-13.64461180448643, "Y"=4020.9353314725367}, {"X"=-10.380186862304981, "Y"=4043.0984315132105}, {"X"=-6.979833146683177, "Y"=4065.2410842048967}, {"X"=-1.4697297999809962, "Y"=4087.0407015995165}, {"X"=2.2000808792763564, "Y"=4109.12785355368}, {"X"=6.005346692003968, "Y"=4131.19207218844}, {"X"=10.929770378021203, "Y"=4153.0535099371555}, {"X"=16.96985273450491, "Y"=4174.693236802181}, {"X"=21.177142139041734, "Y"=4196.665595570732}, {"X"=25.51917220141786, "Y"=4218.611725273365}, {"X"=29.995779446655888, "Y"=4240.530799650704}, {"X"=34.606795333023456, "Y"=4262.421993461985}, {"X"=39.35204625837832, "Y"=4284.2844825161355}, {"X"=44.23135356670491, "Y"=4306.117443702798}, {"X"=50.2184105341189, "Y"=4327.69297876029}, {"X"=54.39139747939407, "Y"=4349.6914956217215}, {"X"=60.64276863692294, "Y"=4371.191935682311}, {"X"=66.05492926119678, "Y"=4392.892623444115}, {"X"=71.60014091999074, "Y"=4414.559694303313}, {"X"=76.31174166907931, "Y"=4436.449175396509}, {"X"=78.26458215041703, "Y"=4459.103564097132}, {"X"=80.36291249774058, "Y"=4481.769205199782}, {"X"=86.453191266457, "Y"=4503.346810847743}, {"X"=92.675753086658, "Y"=4524.88664105537}, {"X"=99.03036368240737, "Y"=4546.387884860228}, {"X"=96.90968228848942, "Y"=4570.479904508192}, {"X"=101.63490128460626, "Y"=4592.550518781641}, {"X"=108.40452097556545, "Y"=4613.995516533227}, {"X"=117.20720403105815, "Y"=4634.778983038918}, {"X"=124.23563956341286, "Y"=4656.127635998224}]}, {"Line"=[{"X"=116.24405358750664, "Y"=4682.575792850332}, {"X"=1470.8259571533572, "Y"=4356.529564736725}, {"X"=1476.1216048608221, "Y"=4369.577807134607}, {"X"=1493.49744902776, "Y"=4377.593871188402}, {"X"=1498.9219181053986, "Y"=4390.502607397701}, {"X"=1938.6303433573366, "Y"=4228.317831710194}, {"X"=1943.130492374914, "Y"=4238.4980939056}, {"X"=2064.2835911828975, "Y"=4195.824052250209}, {"X"=2157.596803563967, "Y"=4164.241687122327}, {"X"=2184.342933978691, "Y"=4162.483261240568}, {"X"=2240.815053624293, "Y"=4146.251716860904}, {"X"=2273.6207227573095, "Y"=4140.661387084596}, {"X"=2307.20330673012, "Y"=4134.252875334802}, {"X"=2353.1869782092754, "Y"=4121.213561259799}, {"X"=2382.006623386713, "Y"=4116.211923388506}, {"X"=2411.6065232364003, "Y"=4110.423577842243}, {"X"=2447.295432626557, "Y"=4101.059215349373}, {"X"=2473.9850587374376, "Y"=4095.9583475826716}, {"X"=2498.805913782341, "Y"=4091.4994374293647}, {"X"=2516.504578766092, "Y"=4090.5875651968613}, {"X"=2551.6517061741442, "Y"=4079.8015650482653}, {"X"=2575.2872437016113, "Y"=4074.968492249235}, {"X"=2594.4778607566627, "Y"=4072.3410062991315}, {"X"=2611.865014281955, "Y"=4070.5}, {"X"=2636.9576668055656, "Y"=4063.91973229833}, {"X"=2659.3520795735667, "Y"=4058.5852574114597}, {"X"=2678.2173574415674, "Y"=4055.061041578305}, {"X"=2691.0289338111706, "Y"=4054.9744145738096}, {"X"=2721.660278831192, "Y"=4043.6987531870027}, {"X"=2739.4124804842736, "Y"=4040.041777322615}, {"X"=2750.3361329295954, "Y"=4040.4815565724384}, {"X"=2767.115634515412, "Y"=4037.014556349579}, {"X"=2782.982986635797, "Y"=4033.9093554840906}, {"X"=2807.9514900820814, "Y"=4024.5561532732263}, {"X"=2814.50634246743, "Y"=4027.177118221292}, {"X"=2830.9861725688024, "Y"=4022.9892285885253}, {"X"=2853.1485517299434, "Y"=4014.6473688040373}, {"X"=2857.1403612634576, "Y"=4018.6478160912407}, {"X"=2872.582789543413, "Y"=4014.533965770538}, {"X"=2885.50776424397, "Y"=4011.997895546798}, {"X"=2893.5183185882197, "Y"=4012.847573680118}, {"X"=2899.900941786414, "Y"=4014.8031747070427}, {"X"=2912.6967434174403, "Y"=4011.9211203798964}, {"X"=2931.0186065410116, "Y"=4004.685937198244}, {"X"=2945.2522496038464, "Y"=4000.2813042191124}, {"X"=2954.661095425663, "Y"=3999.3933301945417}, {"X"=2967.182500916552, "Y"=3995.94154177057}, {"X"=2976.503747613994, "Y"=3994.8418164025816}, {"X"=2988.905267857863, "Y"=3991.1407418939402}, {"X"=2993.4815525575614, "Y"=3993.618651300793}, {"X"=3003.4671589723284, "Y"=3991.6071292968145}, {"X"=3015.7083674570613, "Y"=3987.569777714234}, {"X"=3022.5302826587013, "Y"=3987.918769421469}, {"X"=3030.0942129466903, "Y"=3987.552452442963}, {"X"=3046.702190705782, "Y"=3979.2551869622475}, {"X"=3057.1716590001784, "Y"=3976.0476785022497}, {"X"=3067.5806510774983, "Y"=3972.729983069553}, {"X"=3074.953442415055, "Y"=3971.9768133798516}, {"X"=3079.338473615689, "Y"=3973.843407618128}, {"X"=3090.3454777343677, "Y"=3969.5756253620816}, {"X"=3094.698855111437, "Y"=3971.3297709399512}, {"X"=3103.4168856555025, "Y"=3968.92879048734}, {"X"=3107.7491971523373, "Y"=3970.584898924553}, {"X"=3123.58038741206, "Y"=3961.0784670113726}, {"X"=3127.132781099316, "Y"=3963.2932044495506}, {"X"=3141.3442900960695, "Y"=3954.9186078547696}, {"X"=3145.5555703671926, "Y"=3956.307199565942}, {"X"=3151.8704643852734, "Y"=3955.5226880296186}, {"X"=3156.0677567657553, "Y"=3956.8294686390223}, {"X"=3159.5716639723732, "Y"=3958.823365603732}, {"X"=3175.4683402686765, "Y"=3947.7296839453106}, {"X"=3178.2235496518883, "Y"=3950.3261328545645}, {"X"=3180.994638680067, "Y"=3952.9056272394423}, {"X"=3195.249435679037, "Y"=3942.9187066289505}, {"X"=3197.974753086856, "Y"=3945.3938715838212}, {"X"=3201.380681173798, "Y"=3947.1058472649793}, {"X"=3206.7751036892987, "Y"=3946.541354099974}, {"X"=3212.803756375196, "Y"=3945.173077491038}, {"X"=3218.8006896511197, "Y"=3943.7477727150167}, {"X"=3224.1184753772477, "Y"=3943.0283054696115}, {"X"=3228.7707174038055, "Y"=3943.026883770178}, {"X"=3236.596467994627, "Y"=3939.1330924970466}, {"X"=3243.09464444919, "Y"=3936.7087899036956}, {"X"=3247.0370537459103, "Y"=3937.33414978896}, {"X"=3255.336482079424, "Y"=3932.453534399492}, {"X"=3258.6149065322234, "Y"=3933.7743860095907}, {"X"=3264.351012075589, "Y"=3931.9129043051607}, {"X"=3269.4425440482646, "Y"=3930.7908637781406}, {"X"=3272.6959317916744, "Y"=3932.0139429859637}, {"X"=3277.1498206927595, "Y"=3931.6118183290196}, {"X"=3284.5566606113143, "Y"=3927.1492709057507}, {"X"=3290.7181866922274, "Y"=3924.2284289826134}, {"X"=3293.3270255400894, "Y"=3926.118160532863}, {"X"=3297.105706031337, "Y"=3926.3614038362584}, {"X"=3304.8947253046604, "Y"=3920.8430548874344}, {"X"=3308.6207253100038, "Y"=3921.001328122765}, {"X"=3311.2094260290082, "Y"=3922.7812725103904}, {"X"=3314.926933145405, "Y"=3922.8869193461956}, {"X"=3318.0809533830084, "Y"=3923.7955298897887}, {"X"=3324.527865814621, "Y"=3919.6654659217893}, {"X"=3329.8261174974987, "Y"=3917.1511395328134}, {"X"=3334.0061420335082, "Y"=3916.2730684587964}, {"X"=3338.165158372983, "Y"=3915.359501769437}, {"X"=3341.2467531813195, "Y"=3916.109068948024}, {"X"=3349.556141722818, "Y"=3908.312225938973}, {"X"=3352.0662129768757, "Y"=3909.8412342021875}, {"X"=3356.12266085134, "Y"=3908.7784772340265}, {"X"=3358.635469356694, "Y"=3910.2671853162724}, {"X"=3361.659135341594, "Y"=3910.875446131651}, {"X"=3366.6669726322425, "Y"=3907.989826269476}, {"X"=3370.1569787062945, "Y"=3907.671663919117}, {"X"=3375.5773121030506, "Y"=3903.8297378315624}, {"X"=3379.9809532133554, "Y"=3901.6909496753647}, {"X"=3381.0248231909495, "Y"=3905.6733562134013}, {"X"=3384.9268861109003, "Y"=3904.360675241852}, {"X"=3387.4120452614275, "Y"=3905.672727084371}, {"X"=3391.740097239402, "Y"=3903.415186751994}, {"X"=3396.9388950941193, "Y"=3899.337185439076}, {"X"=3399.3930045680063, "Y"=3900.5756275458457}, {"X"=3402.2969554721067, "Y"=3900.902115465112}, {"X"=3404.7605663121444, "Y"=3902.107651672093}, {"X"=3407.231527806511, "Y"=3903.2980487532614}, {"X"=3410.1354521890526, "Y"=3903.5684000074143}, {"X"=3415.9764364638286, "Y"=3897.4661344862584}, {"X"=3419.2478453327217, "Y"=3896.7677640423126}, {"X"=3421.685769173619, "Y"=3897.8693693724063}, {"X"=3424.1304064445235, "Y"=3898.9559951456195}, {"X"=3428.570407478858, "Y"=3895.4401279688686}, {"X"=3431.000009603355, "Y"=3896.484556125373}, {"X"=3434.595352849846, "Y"=3894.747137673135}, {"X"=3437.0205894479313, "Y"=3895.754610505172}, {"X"=3440.2021866047417, "Y"=3894.893224598871}, {"X"=3442.997631366253, "Y"=3894.937028199931}, {"X"=3445.7875834697406, "Y"=3894.9614292407523}, {"X"=3447.855938217865, "Y"=3896.8339507456913}, {"X"=3453.1117300168457, "Y"=3890.272771457805}, {"X"=3455.509163854388, "Y"=3891.166714164104}, {"X"=3457.912037690245, "Y"=3892.0459296647036}, {"X"=3460.9901878630535, "Y"=3891.0259225801415}, {"X"=3465.367148692672, "Y"=3886.2058976101466}, {"X"=3467.7393979566095, "Y"=3887.0247190388745}, {"X"=3470.7517532769834, "Y"=3885.9324950286336}, {"X"=3473.433962618886, "Y"=3885.7681145217193}, {"X"=3475.497470820703, "Y"=3887.489509829567}, {"X"=3479.0776275398593, "Y"=3884.430461642429}, {"X"=3482.0271182627307, "Y"=3883.2537007970104}, {"X"=3483.804285900354, "Y"=3885.8854182589353}, {"X"=3486.7391138662306, "Y"=3884.672551233115}, {"X"=3490.4843260336584, "Y"=3880.555274770562}, {"X"=3492.821430903891, "Y"=3881.2200864677916}, {"X"=3494.6330890219583, "Y"=3883.7991845626375}, {"X"=3497.507658139402, "Y"=3882.506627210471}, {"X"=3499.8566040708733, "Y"=3883.1283078183887}, {"X"=3502.9501588268386, "Y"=3880.828476257047}, {"X"=3505.2887053640984, "Y"=3881.4167938992614}, {"X"=3507.6308177280707, "Y"=3881.9907514147626}, {"X"=3510.434543069118, "Y"=3880.603506190842}, {"X"=3513.2177495607757, "Y"=3879.196309328959}, {"X"=3516.631613886397, "Y"=3874.8409158520626}, {"X"=3518.9331638941576, "Y"=3875.3453983783315}, {"X"=3521.6479859911105, "Y"=3873.8782715012344}, {"X"=3524.1426355863878, "Y"=3873.3720132310673}, {"X"=3526.241947276591, "Y"=3874.81161889468}, {"X"=3528.54313660979, "Y"=3875.257134075334}, {"X"=3530.847016253508, "Y"=3875.6885210369855}, {"X"=3532.2785452725334, "Y"=3881.0286138462516}, {"X"=3534.6177677323685, "Y"=3881.4369721247554}, {"X"=3537.448138216478, "Y"=3878.8710395205935}, {"X"=3540.244540164776, "Y"=3876.284845588925}, {"X"=3542.554505452179, "Y"=3876.644414741751}, {"X"=3545.879582520246, "Y"=3870.0634815971675}, {"X"=3548.2899011305954, "Y"=3869.3982480669288}, {"X"=3550.5574595983317, "Y"=3869.7085814511606}, {"X"=3552.953349041593, "Y"=3869.013025018898}, {"X"=3555.459217026101, "Y"=3867.3092956243718}, {"X"=3557.713822962267, "Y"=3867.5756782371946}, {"X"=3560.1863992142376, "Y"=3865.839961174927}, {"X"=3562.4319004958415, "Y"=3866.0773660029336}, {"X"=3564.486853239697, "Y"=3868.291754465371}, {"X"=3566.657445372384, "Y"=3869.498679362869}, {"X"=3568.9252743111374, "Y"=3869.696309723754}, {"X"=3571.1942731957497, "Y"=3869.880021227531}, {"X"=3573.4643565996953, "Y"=3870.049806957566}, {"X"=3575.9970515725377, "Y"=3866.2142248285672}, {"X"=3578.4223891140427, "Y"=3863.359885937419}, {"X"=3580.7586355337407, "Y"=3861.4882707550505}, {"X"=3582.9770480783645, "Y"=3861.5995286333678}, {"X"=3585.196101527507, "Y"=3861.697172493809}, {"X"=3587.346185883872, "Y"=3863.779989812956}, {"X"=3589.5785361435096, "Y"=3863.850784101241}, {"X"=3591.811278765371, "Y"=3863.9078796131535}, {"X"=3594.044329687959, "Y"=3863.9512741990807}, {"X"=3596.2776048381675, "Y"=3863.9809662252396}, {"X"=3598.5232919465293, "Y"=3860.9969796734104}, {"X"=3600.734264958528, "Y"=3858.999249100845}, {"X"=3602.9124856990015, "Y"=3855.988086074595}, {"X"=3605.1110493698097, "Y"=3856.963411534487}, {"X"=3607.301239472894, "Y"=3856.9253309897736}, {"X"=3609.491154688439, "Y"=3856.8738124080837}, {"X"=3611.680712567374, "Y"=3856.8088577290628}, {"X"=3613.869830674083, "Y"=3856.730469398217}, {"X"=3616.0584265895063, "Y"=3856.6386503668236}, {"X"=3618.144197085594, "Y"=3854.5360180744956}, {"X"=3620.262010319799, "Y"=3853.4196527328386}, {"X"=3622.4301711150943, "Y"=3853.2886743496706}, {"X"=3624.5974874271237, "Y"=3853.1443948475926}, {"X"=3626.7638776576546, "Y"=3852.9868196586467}, {"X"=3628.847539169185, "Y"=3851.8192994761407}, {"X"=3631.0057187613443, "Y"=3851.6356714044987}, {"X"=3633.068785592103, "Y"=3850.4432270988605}, {"X"=3635.3184946920105, "Y"=3851.2287060202943}, {"X"=3637.3667730516813, "Y"=3850.01103449992}, {"X"=3639.513696966361, "Y"=3849.775167431953}, {"X"=3641.6591332126836, "Y"=3849.5261315266252}, {"X"=3643.803001016186, "Y"=3849.263936159999}, {"X"=3645.9452196614584, "Y"=3848.988591203581}, {"X"=3648.358922747992, "Y"=3850.681357632044}, {"X"=3650.5097527639764, "Y"=3850.3780313828506}, {"X"=3652.658681116318, "Y"=3850.06151359881}, {"X"=3654.805626899078, "Y"=3849.731816196638}, {"X"=3656.9505092809613, "Y"=3849.3889515892556}, {"X"=3659.093247508359, "Y"=3849.0329326853207}, {"X"=3661.233760908388, "Y"=3848.663772888745}, {"X"=3663.371968891928, "Y"=3848.2814860981853}, {"X"=3665.507790956657, "Y"=3847.8860867065237}, {"X"=3667.6411466900818, "Y"=3847.4775896003234}, {"X"=3669.771955772565, "Y"=3847.05601015927}, {"X"=3672.3063534491635, "Y"=3848.579677047995}, {"X"=3674.6529488935626, "Y"=3849.107343408149}, {"X"=3676.7936259622215, "Y"=3848.642709677937}, {"X"=3678.931411794267, "Y"=3848.1649497467597}, {"X"=3681.9745309554087, "Y"=3851.5695895191175}, {"X"=3682.265797573908, "Y"=3843.2802623943426}, {"X"=3684.3705770359, "Y"=3842.7690267959306}, {"X"=3685.982252627952, "Y"=3840.3058216266995}, {"X"=3689.072343340926, "Y"=3843.6438820228814}, {"X"=3690.408697130985, "Y"=3840.191515889326}, {"X"=3692.7571392126815, "Y"=3840.5952335618913}, {"X"=3694.845246150937, "Y"=3840.019674846277}, {"X"=3696.929782219281, "Y"=3839.4313145820856}, {"X"=3699.01066893611, "Y"=3838.830174920747}, {"X"=3701.0878279572144, "Y"=3838.2162784948305}, {"X"=3702.868939772559, "Y"=3836.6333038041093}, {"X"=3704.336338764959, "Y"=3834.086707926436}, {"X"=3706.9922024064654, "Y"=3835.3455958026198}, {"X"=3707.4988553411154, "Y"=3829.928774283708}, {"X"=3709.5212366069845, "Y"=3829.262962891481}, {"X"=3712.1823733908036, "Y"=3830.478615193792}, {"X"=3714.8625275878517, "Y"=3831.6739359011044}, {"X"=3716.8954783450504, "Y"=3830.9629090132034}, {"X"=3718.9240280535587, "Y"=3830.239421558839}, {"X"=3721.9818447869743, "Y"=3832.3197700143137}, {"X"=3725.069629579242, "Y"=3834.3749209449047}, {"X"=3726.0507345592364, "Y"=3830.79784206835}, {"X"=3728.078099090901, "Y"=3830.01818212526}, {"X"=3730.1006415545253, "Y"=3829.22609718414}, {"X"=3731.7450703059103, "Y"=3827.493872385562}, {"X"=3732.994252855881, "Y"=3824.8284604330506}, {"X"=3734.984859240635, "Y"=3824.006308234556}, {"X"=3737.750841547497, "Y"=3825.0133930362813}, {"X"=3741.3259774571916, "Y"=3827.8352758562896}, {"X"=3743.3348764721827, "Y"=3826.9619445542617}, {"X"=3745.338379010088, "Y"=3826.0763033198214}, {"X"=3747.3364096401688, "Y"=3825.17838549686}, {"X"=3749.747181353774, "Y"=3825.176539246914}, {"X"=3751.739608140834, "Y"=3824.2515864591355}, {"X"=3753.7263220174113, "Y"=3823.314425782394}, {"X"=3755.707248184851, "Y"=3822.3650925002603}, {"X"=3758.563218833701, "Y"=3823.19917331747}, {"X"=3760.989300513128, "Y"=3823.1152195739064}, {"X"=3762.5174303442213, "Y"=3821.229022403504}, {"X"=3764.9422991025817, "Y"=3821.11530322729}, {"X"=3766.909520570095, "Y"=3820.0971914013944}, {"X"=3770.273813595049, "Y"=3821.718554646446}, {"X"=3772.244636179431, "Y"=3820.6677179065823}, {"X"=3774.208973850614, "Y"=3819.604808208381}, {"X"=3775.1988034619967, "Y"=3816.779701473255}, {"X"=3776.1605593274253, "Y"=3813.95454661057}, {"X"=3778.083632037759, "Y"=3812.8677356331905}, {"X"=3781.0, "Y"=3813.5011961699665}]}]
  in  "min line size":i32=20
  out "split":cluster{"Line":cluster{"X":dbl, "Y":dbl}[]}[](graph)=[{"Line"=[{"X"=4702.197140342376, "Y"=1516.6890148488842}, {"X"=4604.143011328081, "Y"=1554.8990224667068}]}, {"Line"=[{"X"=4592.189193390564, "Y"=1548.7743327541575}, {"X"=4594.527091192987, "Y"=1514.1105607604393}, {"X"=4582.323180976402, "Y"=1508.045641055899}, {"X"=4580.564941005001, "Y"=1480.4660447341178}, {"X"=4571.173600402096, "Y"=1468.1717991222706}, {"X"=4570.608002262242, "Y"=1436.9149057916925}, {"X"=4568.854651859388, "Y"=1407.4043239148123}, {"X"=4555.996487758588, "Y"=1401.4989360514387}, {"X"=4548.828017241294, "Y"=1382.8969336147202}, {"X"=4541.87041502761, "Y"=1363.3893379242631}, {"X"=4537.493154460165, "Y"=1337.4654718732627}, {"X"=4530.088114201489, "Y"=1317.9550646650014}, {"X"=4520.932883548637, "Y"=1302.1438573012124}, {"X"=4510.476099602794, "Y"=1289.1372109395656}, {"X"=4513.398299571488, "Y"=1242.805159863262}, {"X"=4500.178610642434, "Y"=1194.5058080875897}]}, {"Line"=[{"X"=4045.262015510834, "Y"=-370.47254705975547}, {"X"=4021.5048604927456, "Y"=-373.1317628736815}, {"X"=3997.731836054895, "Y"=-375.64515746583857}, {"X"=3974.4237446268694, "Y"=-382.9895518092235}, {"X"=3948.973422153729, "Y"=-367.28671688954455}, {"X"=3924.2325152064327, "Y"=-357.3973448535103}, {"X"=3900.4802229985116, "Y"=-358.3172025621179}, {"X"=3876.8003772484603, "Y"=-360.08828281881506}, {"X"=3852.848497603733, "Y"=-357.72259724044125}, {"X"=3829.173196937117, "Y"=-359.2014259177531}, {"X"=3805.4892680291655, "Y"=-360.5349578426094}, {"X"=3782.314874586134, "Y"=-372.7109737888577}, {"X"=3758.6307242397825, "Y"=-375.7550610593494}, {"X"=3734.846552078191, "Y"=-376.65544089136483}, {"X"=3711.0000422297094, "Y"=-375.4106867047012}, {"X"=3687.3538586650116, "Y"=-382.0172981809769}, {"X"=3662.9108581038413, "Y"=-344.48530026226535}, {"X"=3639.320355486937, "Y"=-344.7989426814479}, {"X"=3615.7774597291873, "Y"=-356.96773019486045}, {"X"=3592.111253634981, "Y"=-356.9919325402784}, {"X"=3568.4453445476156, "Y"=-356.8709213194161}, {"X"=3543.4634903042615, "Y"=-448.5952721279782}, {"X"=3519.2364294721056, "Y"=-448.174039435899}]}, {"Line"=[{"X"=3495.0124093427307, "Y"=-447.6041602227524}, {"X"=3447.5484157840283, "Y"=-421.03742834342756}, {"X"=3429.4298217719656, "Y"=-288.161798854328}, {"X"=3406.547081777543, "Y"=-280.0530377801865}, {"X"=3383.3567540665535, "Y"=-278.7948745587423}, {"X"=3360.744841438998, "Y"=-268.4125263964861}, {"X"=3337.6268007773465, "Y"=-266.8735450409895}, {"X"=3312.0237005706044, "Y"=-298.09829401069464}, {"X"=3288.724428624859, "Y"=-296.2598065286679}, {"X"=3270.706969868897, "Y"=-234.51028922227988}, {"X"=3249.771498047274, "Y"=-211.51235972884115}, {"X"=3227.8050984298025, "Y"=-201.33367250848505}]}, {"Line"=[{"X"=3206.375015694224, "Y"=-187.04805660711145}, {"X"=3183.7591240020847, "Y"=-184.5634114706845}, {"X"=3161.3956031641924, "Y"=-179.95410067521016}, {"X"=3138.8240858920867, "Y"=-177.1936005936277}, {"X"=3116.9225625935896, "Y"=-169.33743194447243}, {"X"=3094.5536322950015, "Y"=-165.31362496769452}, {"X"=3072.0732055742583, "Y"=-162.14326586595462}, {"X"=3050.50517501786, "Y"=-152.90178314690638}, {"X"=3029.3402803672284, "Y"=-141.5578375729042}, {"X"=3005.7198268817183, "Y"=-145.8835795782761}, {"X"=2983.360292949494, "Y"=-142.16851225868822}, {"X"=2961.369928605174, "Y"=-136.34646752894514}, {"X"=2939.069748166673, "Y"=-132.35945388277014}, {"X"=2916.0542503508345, "Y"=-132.16660019014535}, {"X"=2893.971646836575, "Y"=-126.92003834235948}, {"X"=2871.7305746338234, "Y"=-122.51965406356612}, {"X"=2849.516921363317, "Y"=-117.98288396725366}, {"X"=2827.3315233565468, "Y"=-113.3098988602519}, {"X"=2805.820540469126, "Y"=-105.57110400824695}, {"X"=2784.596507850818, "Y"=-96.72922875644326}, {"X"=2761.6344368770942, "Y"=-95.5538074919159}, {"X"=2738.656125118518, "Y"=-94.23186914869939}, {"X"=2716.6185475221346, "Y"=-88.87910208996846}, {"X"=2694.614228738148, "Y"=-83.39121576148591}, {"X"=2672.6439972167227, "Y"=-77.76841677907123}, {"X"=2650.708680124659, "Y"=-72.01091683792765}, {"X"=2628.809103314247, "Y"=-66.11893270467408}, {"X"=2606.946091292176, "Y"=-60.092686209182375}, {"X"=2584.5712899521213, "Y"=-55.85552783159346}, {"X"=2561.650151837172, "Y"=-53.3974718317445}, {"X"=2539.293725910705, "Y"=-48.87562477295114}, {"X"=2517.538201938755, "Y"=-42.30044684778477}, {"X"=2494.034809091436, "Y"=-41.3191040202214}, {"X"=2472.0225479250194, "Y"=-35.41905120318597}, {"X"=2450.0410633250167, "Y"=-29.382161789984366}, {"X"=2426.5130901879893, "Y"=-27.95301449719682}, {"X"=2404.2451890722396, "Y"=-22.58008172179325}, {"X"=2382.6535537697796, "Y"=-15.176756558716079}, {"X"=2359.4425731187703, "Y"=-12.355658331004179}, {"X"=2337.9145170954243, "Y"=-4.677621956337134}, {"X"=2315.0556519473794, "Y"=-0.6226620999336774}, {"X"=2293.6004238067435, "Y"=7.327506432634436}, {"X"=2270.057927743648, "Y"=9.802429024614412}, {"X"=2247.5821062096375, "Y"=15.231737897677704}, {"X"=2224.75536526262, "Y"=19.875548974426238}, {"X"=2200.815103181707, "Y"=21.88519100999474}, {"X"=2173.8166160981887, "Y"=16.65434452990621}, {"X"=2150.9317674680565, "Y"=21.778434678614303}, {"X"=2099.569445467065, "Y"=-40.16004596176299}, {"X"=1993.354962067471, "Y"=11.164560761459143}, {"X"=1971.9781148912214, "Y"=21.088425727543836}, {"X"=1946.7979336116412, "Y"=23.015253457493145}, {"X"=1925.494677341689, "Y"=33.224563893850245}, {"X"=1904.2544652507022, "Y"=43.564396465946174}, {"X"=1877.726652128255, "Y"=43.29368976613068}, {"X"=1842.55456574985, "Y"=26.26504384210375}, {"X"=1829.0405780564897, "Y"=52.23569166488596}, {"X"=1814.3917771697875, "Y"=75.5807390798177}, {"X"=1786.8645563340388, "Y"=74.22769832520271}, {"X"=1765.8785444190275, "Y"=85.41737745628188}, {"X"=1747.8331626322108, "Y"=102.00382481748511}, {"X"=1728.9542149611082, "Y"=116.9328013933573}, {"X"=1706.27398723018, "Y"=124.98862393636955}, {"X"=1685.60095559409, "Y"=136.67184194320134}, {"X"=1655.000000000001, "Y"=131.16117927853338}, {"X"=1628.3021546343343, "Y"=132.80359845458497}, {"X"=1607.6785425781395, "Y"=144.9650955174202}, {"X"=1587.1299402987506, "Y"=157.25290774813675}, {"X"=1566.6571214394316, "Y"=169.66657251754714}, {"X"=1546.2608567902394, "Y"=182.2056224581911}, {"X"=1525.9419142590123, "Y"=194.86958548192388}, {"X"=1494.9665691389255, "Y"=190.7828335152658}, {"X"=1455.735015665709, "Y"=174.34567686930814}, {"X"=1430.993243345882, "Y"=180.86838320792322}, {"X"=1410.668265549114, "Y"=194.23964018468632}, {"X"=1390.425714854734, "Y"=207.7353571705712}, {"X"=1357.3322111709276, "Y"=202.3364045208432}, {"X"=1334.8706766640394, "Y"=212.86551103190004}, {"X"=1311.3090852839077, "Y"=221.9063623965808}, {"X"=1275.0687472590512, "Y"=213.15186386282812}, {"X"=1254.9447924102292, "Y"=227.47924783415692}, {"X"=1234.9091275645433, "Y"=241.92984036216785}]}, {"Line"=[{"X"=713.0611631530592, "Y"=-278.30771011372644}, {"X"=573.1977201747654, "Y"=410.6484565778592}]}, {"Line"=[{"X"=592.3260462109588, "Y"=467.61836377757436}, {"X"=573.776320891091, "Y"=486.13018794763866}, {"X"=516.8456561375579, "Y"=466.8853810114342}, {"X"=481.7982266209283, "Y"=469.8314072488288}, {"X"=435.128765874887, "Y"=462.0139777465424}, {"X"=416.5476118831816, "Y"=481.49045179689256}, {"X"=381.2994394025459, "Y"=485.35794807913635}, {"X"=362.86253464191304, "Y"=505.1642732238183}, {"X"=342.3329127440702, "Y"=523.0595994193186}, {"X"=336.7475675292044, "Y"=554.4950242830287}]}, {"Line"=[{"X"=270.96481001367874, "Y"=531.983035117094}, {"X"=568.1778192565093, "Y"=1887.4212377834735}, {"X"=558.3402951796288, "Y"=1906.0545053007447}, {"X"=548.617287871481, "Y"=1924.7477839649912}, {"X"=532.7695198753122, "Y"=1940.3275402206798}, {"X"=529.5162834990319, "Y"=1962.3115573360112}, {"X"=539.8702058904678, "Y"=1990.9109889727677}, {"X"=605.3325001870285, "Y"=2045.968512870534}, {"X"=601.8805011027116, "Y"=2066.9583152148466}, {"X"=605.8120277476805, "Y"=2091.3412809272986}, {"X"=674.3588639641607, "Y"=2145.452125934663}, {"X"=666.1025888247354, "Y"=2163.429021451132}, {"X"=657.9567732645942, "Y"=2181.4562381095116}, {"X"=619.7255133273352, "Y"=2186.221866490394}, {"X"=604.3804690989409, "Y"=2201.3512306693083}, {"X"=596.4685017416655, "Y"=2219.7564532597535}, {"X"=596.0480668191567, "Y"=2241.301551943805}, {"X"=707.6625662145384, "Y"=2308.879448114789}, {"X"=715.2401057472161, "Y"=2332.650715290977}, {"X"=717.4243259383866, "Y"=2354.0674176426273}, {"X"=719.7624075179106, "Y"=2375.413226623674}, {"X"=726.9221966011937, "Y"=2398.476992697342}, {"X"=720.2174633677091, "Y"=2416.1266025463633}, {"X"=715.4972516675775, "Y"=2434.5100212284015}, {"X"=731.5776225251552, "Y"=2460.4067793595614}, {"X"=730.9061825143826, "Y"=2480.0364386578276}, {"X"=719.9804701443845, "Y"=2496.014189517481}, {"X"=750.778902136793, "Y"=2526.316203538756}, {"X"=755.2887344326768, "Y"=2547.3102207148654}, {"X"=758.99836842379, "Y"=2567.9003650996783}, {"X"=769.5176591565032, "Y"=2590.550321252946}, {"X"=776.3916464972967, "Y"=2611.8356762232834}, {"X"=797.7559831999147, "Y"=2637.415238768894}, {"X"=794.4310781670474, "Y"=2655.202376397113}, {"X"=807.5266916718274, "Y"=2677.7994026548567}, {"X"=802.5343311689248, "Y"=2694.949174454491}, {"X"=797.6472936673199, "Y"=2712.1292559626913}, {"X"=792.8657631612118, "Y"=2729.3390003590985}, {"X"=738.9277025317801, "Y"=2733.377988406333}]}, {"Line"=[{"X"=734.2776571765958, "Y"=2750.94762943921}, {"X"=804.3507531766409, "Y"=2787.56032624791}, {"X"=811.678247143569, "Y"=2807.6194669492497}, {"X"=814.2862759422133, "Y"=2826.386574067813}, {"X"=836.487585483886, "Y"=2849.676899675769}, {"X"=853.0200522133496, "Y"=2871.330638206337}, {"X"=849.2143206481433, "Y"=2888.19762482257}, {"X"=849.4220025087889, "Y"=2905.932091661871}, {"X"=845.8286492029479, "Y"=2922.82050413347}, {"X"=842.3389888918005, "Y"=2939.7306470868652}, {"X"=844.8402464495775, "Y"=2957.8203873106486}, {"X"=851.3888451759594, "Y"=2976.606534644484}, {"X"=857.0804053085021, "Y"=2995.110807149304}, {"X"=861.9106586397288, "Y"=3013.350476493323}, {"X"=892.4874355899142, "Y"=3035.904413335442}, {"X"=1025.8475465905508, "Y"=3075.0057099135174}, {"X"=1023.2882883425077, "Y"=3090.8084128343826}]}, {"Line"=[{"X"=1304.545062912477, "Y"=3149.899111968396}, {"X"=1302.4400955384413, "Y"=3163.990349229975}]}, {"Line"=[{"X"=914.1062820436955, "Y"=3224.364487333619}, {"X"=933.3686210466781, "Y"=3242.8656211598604}, {"X"=941.800605877364, "Y"=3260.131325333941}, {"X"=940.3788392110519, "Y"=3276.4462456507435}, {"X"=939.0572057782192, "Y"=3292.769582640043}, {"X"=948.8075824980851, "Y"=3309.887492835553}, {"X"=950.6845588015076, "Y"=3326.35469189397}, {"X"=952.6636881702325, "Y"=3342.7916921165966}, {"X"=952.7474978684022, "Y"=3359.091554695986}, {"X"=954.9294148586805, "Y"=3375.478517435108}, {"X"=960.2101388711521, "Y"=3391.956077999096}, {"X"=971.5896340437512, "Y"=3408.572716688413}, {"X"=974.0768960605492, "Y"=3424.7879517829642}, {"X"=981.6628112449193, "Y"=3441.081700787105}, {"X"=981.3505848148575, "Y"=3457.1486248702304}, {"X"=993.1363215681313, "Y"=3473.3398786074254}, {"X"=994.0218032440225, "Y"=3489.3398859076315}, {"X"=1020.0053964340373, "Y"=3505.2768902312037}, {"X"=1022.0862755609401, "Y"=3521.09097789895}, {"X"=1022.2642158658068, "Y"=3536.908362115882}, {"X"=1025.5385789953302, "Y"=3552.663001800286}, {"X"=1025.91017660836, "Y"=3568.4586087471434}, {"X"=1014.3851121986418, "Y"=3584.6442672599346}, {"X"=975.9825976478487, "Y"=3602.0229001404546}, {"X"=947.6873481122784, "Y"=3619.426113711875}, {"X"=927.497508824365, "Y"=3636.771468735349}, {"X"=928.3870318839645, "Y"=3653.1670610615342}, {"X"=905.4253651296312, "Y"=3671.0775763015645}, {"X"=1015.481200145904, "Y"=3743.8822937417594}, {"X"=1026.9761083045855, "Y"=3758.735488027024}, {"X"=1028.6121158613832, "Y"=3774.518395203543}, {"X"=1030.3449347186652, "Y"=3790.29096691764}, {"X"=1029.195583743087, "Y"=3806.4076587716963}, {"X"=1031.1240604595514, "Y"=3822.1760500878013}]}, {"Line"=[{"X"=-10.842185123417494, "Y"=3975.376392065428}, {"X"=-7.85735733306592, "Y"=3997.523154373408}, {"X"=-13.64461180448643, "Y"=4020.9353314725367}, {"X"=-10.380186862304981, "Y"=4043.0984315132105}, {"X"=-6.979833146683177, "Y"=4065.2410842048967}, {"X"=-1.4697297999809962, "Y"=4087.0407015995165}, {"X"=2.2000808792763564, "Y"=4109.12785355368}, {"X"=6.005346692003968, "Y"=4131.19207218844}, {"X"=10.929770378021203, "Y"=4153.0535099371555}, {"X"=16.96985273450491, "Y"=4174.693236802181}, {"X"=21.177142139041734, "Y"=4196.665595570732}, {"X"=25.51917220141786, "Y"=4218.611725273365}, {"X"=29.995779446655888, "Y"=4240.530799650704}, {"X"=34.606795333023456, "Y"=4262.421993461985}, {"X"=39.35204625837832, "Y"=4284.2844825161355}, {"X"=44.23135356670491, "Y"=4306.117443702798}, {"X"=50.2184105341189, "Y"=4327.69297876029}, {"X"=54.39139747939407, "Y"=4349.6914956217215}, {"X"=60.64276863692294, "Y"=4371.191935682311}, {"X"=66.05492926119678, "Y"=4392.892623444115}, {"X"=71.60014091999074, "Y"=4414.559694303313}, {"X"=76.31174166907931, "Y"=4436.449175396509}, {"X"=78.26458215041703, "Y"=4459.103564097132}, {"X"=80.36291249774058, "Y"=4481.769205199782}, {"X"=86.453191266457, "Y"=4503.346810847743}, {"X"=92.675753086658, "Y"=4524.88664105537}, {"X"=99.03036368240737, "Y"=4546.387884860228}, {"X"=96.90968228848942, "Y"=4570.479904508192}, {"X"=101.63490128460626, "Y"=4592.550518781641}, {"X"=108.40452097556545, "Y"=4613.995516533227}, {"X"=117.20720403105815, "Y"=4634.778983038918}, {"X"=124.23563956341286, "Y"=4656.127635998224}]}, {"Line"=[{"X"=116.24405358750664, "Y"=4682.575792850332}, {"X"=1470.8259571533572, "Y"=4356.529564736725}, {"X"=1476.1216048608221, "Y"=4369.577807134607}, {"X"=1493.49744902776, "Y"=4377.593871188402}, {"X"=1498.9219181053986, "Y"=4390.502607397701}, {"X"=1938.6303433573366, "Y"=4228.317831710194}, {"X"=1943.130492374914, "Y"=4238.4980939056}, {"X"=2064.2835911828975, "Y"=4195.824052250209}, {"X"=2157.596803563967, "Y"=4164.241687122327}, {"X"=2184.342933978691, "Y"=4162.483261240568}, {"X"=2240.815053624293, "Y"=4146.251716860904}, {"X"=2273.6207227573095, "Y"=4140.661387084596}, {"X"=2307.20330673012, "Y"=4134.252875334802}, {"X"=2353.1869782092754, "Y"=4121.213561259799}, {"X"=2382.006623386713, "Y"=4116.211923388506}, {"X"=2411.6065232364003, "Y"=4110.423577842243}, {"X"=2447.295432626557, "Y"=4101.059215349373}, {"X"=2473.9850587374376, "Y"=4095.9583475826716}, {"X"=2498.805913782341, "Y"=4091.4994374293647}, {"X"=2516.504578766092, "Y"=4090.5875651968613}, {"X"=2551.6517061741442, "Y"=4079.8015650482653}, {"X"=2575.2872437016113, "Y"=4074.968492249235}, {"X"=2594.4778607566627, "Y"=4072.3410062991315}, {"X"=2611.865014281955, "Y"=4070.5}, {"X"=2636.9576668055656, "Y"=4063.91973229833}, {"X"=2659.3520795735667, "Y"=4058.5852574114597}, {"X"=2678.2173574415674, "Y"=4055.061041578305}, {"X"=2691.0289338111706, "Y"=4054.9744145738096}, {"X"=2721.660278831192, "Y"=4043.6987531870027}, {"X"=2739.4124804842736, "Y"=4040.041777322615}, {"X"=2750.3361329295954, "Y"=4040.4815565724384}, {"X"=2767.115634515412, "Y"=4037.014556349579}, {"X"=2782.982986635797, "Y"=4033.9093554840906}, {"X"=2807.9514900820814, "Y"=4024.5561532732263}, {"X"=2814.50634246743, "Y"=4027.177118221292}, {"X"=2830.9861725688024, "Y"=4022.9892285885253}, {"X"=2853.1485517299434, "Y"=4014.6473688040373}, {"X"=2857.1403612634576, "Y"=4018.6478160912407}, {"X"=2872.582789543413, "Y"=4014.533965770538}, {"X"=2885.50776424397, "Y"=4011.997895546798}, {"X"=2893.5183185882197, "Y"=4012.847573680118}, {"X"=2899.900941786414, "Y"=4014.8031747070427}, {"X"=2912.6967434174403, "Y"=4011.9211203798964}, {"X"=2931.0186065410116, "Y"=4004.685937198244}, {"X"=2945.2522496038464, "Y"=4000.2813042191124}, {"X"=2954.661095425663, "Y"=3999.3933301945417}, {"X"=2967.182500916552, "Y"=3995.94154177057}, {"X"=2976.503747613994, "Y"=3994.8418164025816}, {"X"=2988.905267857863, "Y"=3991.1407418939402}, {"X"=2993.4815525575614, "Y"=3993.618651300793}, {"X"=3003.4671589723284, "Y"=3991.6071292968145}, {"X"=3015.7083674570613, "Y"=3987.569777714234}, {"X"=3022.5302826587013, "Y"=3987.918769421469}, {"X"=3030.0942129466903, "Y"=3987.552452442963}, {"X"=3046.702190705782, "Y"=3979.2551869622475}, {"X"=3057.1716590001784, "Y"=3976.0476785022497}, {"X"=3067.5806510774983, "Y"=3972.729983069553}, {"X"=3074.953442415055, "Y"=3971.9768133798516}, {"X"=3079.338473615689, "Y"=3973.843407618128}, {"X"=3090.3454777343677, "Y"=3969.5756253620816}, {"X"=3094.698855111437, "Y"=3971.3297709399512}, {"X"=3103.4168856555025, "Y"=3968.92879048734}, {"X"=3107.7491971523373, "Y"=3970.584898924553}, {"X"=3123.58038741206, "Y"=3961.0784670113726}, {"X"=3127.132781099316, "Y"=3963.2932044495506}, {"X"=3141.3442900960695, "Y"=3954.9186078547696}, {"X"=3145.5555703671926, "Y"=3956.307199565942}, {"X"=3151.8704643852734, "Y"=3955.5226880296186}, {"X"=3156.0677567657553, "Y"=3956.8294686390223}, {"X"=3159.5716639723732, "Y"=3958.823365603732}, {"X"=3175.4683402686765, "Y"=3947.7296839453106}, {"X"=3178.2235496518883, "Y"=3950.3261328545645}, {"X"=3180.994638680067, "Y"=3952.9056272394423}, {"X"=3195.249435679037, "Y"=3942.9187066289505}, {"X"=3197.974753086856, "Y"=3945.3938715838212}, {"X"=3201.380681173798, "Y"=3947.1058472649793}, {"X"=3206.7751036892987, "Y"=3946.541354099974}, {"X"=3212.803756375196, "Y"=3945.173077491038}, {"X"=3218.8006896511197, "Y"=3943.7477727150167}, {"X"=3224.1184753772477, "Y"=3943.0283054696115}, {"X"=3228.7707174038055, "Y"=3943.026883770178}, {"X"=3236.596467994627, "Y"=3939.1330924970466}, {"X"=3243.09464444919, "Y"=3936.7087899036956}, {"X"=3247.0370537459103, "Y"=3937.33414978896}, {"X"=3255.336482079424, "Y"=3932.453534399492}, {"X"=3258.6149065322234, "Y"=3933.7743860095907}, {"X"=3264.351012075589, "Y"=3931.9129043051607}, {"X"=3269.4425440482646, "Y"=3930.7908637781406}, {"X"=3272.6959317916744, "Y"=3932.0139429859637}, {"X"=3277.1498206927595, "Y"=3931.6118183290196}, {"X"=3284.5566606113143, "Y"=3927.1492709057507}, {"X"=3290.7181866922274, "Y"=3924.2284289826134}, {"X"=3293.3270255400894, "Y"=3926.118160532863}, {"X"=3297.105706031337, "Y"=3926.3614038362584}, {"X"=3304.8947253046604, "Y"=3920.8430548874344}, {"X"=3308.6207253100038, "Y"=3921.001328122765}, {"X"=3311.2094260290082, "Y"=3922.7812725103904}, {"X"=3314.926933145405, "Y"=3922.8869193461956}, {"X"=3318.0809533830084, "Y"=3923.7955298897887}, {"X"=3324.527865814621, "Y"=3919.6654659217893}, {"X"=3329.8261174974987, "Y"=3917.1511395328134}, {"X"=3334.0061420335082, "Y"=3916.2730684587964}, {"X"=3338.165158372983, "Y"=3915.359501769437}, {"X"=3341.2467531813195, "Y"=3916.109068948024}, {"X"=3349.556141722818, "Y"=3908.312225938973}, {"X"=3352.0662129768757, "Y"=3909.8412342021875}, {"X"=3356.12266085134, "Y"=3908.7784772340265}, {"X"=3358.635469356694, "Y"=3910.2671853162724}, {"X"=3361.659135341594, "Y"=3910.875446131651}, {"X"=3366.6669726322425, "Y"=3907.989826269476}, {"X"=3370.1569787062945, "Y"=3907.671663919117}, {"X"=3375.5773121030506, "Y"=3903.8297378315624}, {"X"=3379.9809532133554, "Y"=3901.6909496753647}, {"X"=3381.0248231909495, "Y"=3905.6733562134013}, {"X"=3384.9268861109003, "Y"=3904.360675241852}, {"X"=3387.4120452614275, "Y"=3905.672727084371}, {"X"=3391.740097239402, "Y"=3903.415186751994}, {"X"=3396.9388950941193, "Y"=3899.337185439076}, {"X"=3399.3930045680063, "Y"=3900.5756275458457}, {"X"=3402.2969554721067, "Y"=3900.902115465112}, {"X"=3404.7605663121444, "Y"=3902.107651672093}, {"X"=3407.231527806511, "Y"=3903.2980487532614}, {"X"=3410.1354521890526, "Y"=3903.5684000074143}, {"X"=3415.9764364638286, "Y"=3897.4661344862584}, {"X"=3419.2478453327217, "Y"=3896.7677640423126}, {"X"=3421.685769173619, "Y"=3897.8693693724063}, {"X"=3424.1304064445235, "Y"=3898.9559951456195}, {"X"=3428.570407478858, "Y"=3895.4401279688686}, {"X"=3431.000009603355, "Y"=3896.484556125373}, {"X"=3434.595352849846, "Y"=3894.747137673135}, {"X"=3437.0205894479313, "Y"=3895.754610505172}, {"X"=3440.2021866047417, "Y"=3894.893224598871}, {"X"=3442.997631366253, "Y"=3894.937028199931}, {"X"=3445.7875834697406, "Y"=3894.9614292407523}, {"X"=3447.855938217865, "Y"=3896.8339507456913}, {"X"=3453.1117300168457, "Y"=3890.272771457805}, {"X"=3455.509163854388, "Y"=3891.166714164104}, {"X"=3457.912037690245, "Y"=3892.0459296647036}, {"X"=3460.9901878630535, "Y"=3891.0259225801415}, {"X"=3465.367148692672, "Y"=3886.2058976101466}, {"X"=3467.7393979566095, "Y"=3887.0247190388745}, {"X"=3470.7517532769834, "Y"=3885.9324950286336}, {"X"=3473.433962618886, "Y"=3885.7681145217193}, {"X"=3475.497470820703, "Y"=3887.489509829567}, {"X"=3479.0776275398593, "Y"=3884.430461642429}, {"X"=3482.0271182627307, "Y"=3883.2537007970104}, {"X"=3483.804285900354, "Y"=3885.8854182589353}, {"X"=3486.7391138662306, "Y"=3884.672551233115}, {"X"=3490.4843260336584, "Y"=3880.555274770562}, {"X"=3492.821430903891, "Y"=3881.2200864677916}, {"X"=3494.6330890219583, "Y"=3883.7991845626375}, {"X"=3497.507658139402, "Y"=3882.506627210471}, {"X"=3499.8566040708733, "Y"=3883.1283078183887}, {"X"=3502.9501588268386, "Y"=3880.828476257047}, {"X"=3505.2887053640984, "Y"=3881.4167938992614}, {"X"=3507.6308177280707, "Y"=3881.9907514147626}, {"X"=3510.434543069118, "Y"=3880.603506190842}, {"X"=3513.2177495607757, "Y"=3879.196309328959}, {"X"=3516.631613886397, "Y"=3874.8409158520626}, {"X"=3518.9331638941576, "Y"=3875.3453983783315}, {"X"=3521.6479859911105, "Y"=3873.8782715012344}, {"X"=3524.1426355863878, "Y"=3873.3720132310673}, {"X"=3526.241947276591, "Y"=3874.81161889468}, {"X"=3528.54313660979, "Y"=3875.257134075334}, {"X"=3530.847016253508, "Y"=3875.6885210369855}, {"X"=3532.2785452725334, "Y"=3881.0286138462516}, {"X"=3534.6177677323685, "Y"=3881.4369721247554}, {"X"=3537.448138216478, "Y"=3878.8710395205935}, {"X"=3540.244540164776, "Y"=3876.284845588925}, {"X"=3542.554505452179, "Y"=3876.644414741751}, {"X"=3545.879582520246, "Y"=3870.0634815971675}, {"X"=3548.2899011305954, "Y"=3869.3982480669288}, {"X"=3550.5574595983317, "Y"=3869.7085814511606}, {"X"=3552.953349041593, "Y"=3869.013025018898}, {"X"=3555.459217026101, "Y"=3867.3092956243718}, {"X"=3557.713822962267, "Y"=3867.5756782371946}, {"X"=3560.1863992142376, "Y"=3865.839961174927}, {"X"=3562.4319004958415, "Y"=3866.0773660029336}, {"X"=3564.486853239697, "Y"=3868.291754465371}, {"X"=3566.657445372384, "Y"=3869.498679362869}, {"X"=3568.9252743111374, "Y"=3869.696309723754}, {"X"=3571.1942731957497, "Y"=3869.880021227531}, {"X"=3573.4643565996953, "Y"=3870.049806957566}, {"X"=3575.9970515725377, "Y"=3866.2142248285672}, {"X"=3578.4223891140427, "Y"=3863.359885937419}, {"X"=3580.7586355337407, "Y"=3861.4882707550505}, {"X"=3582.9770480783645, "Y"=3861.5995286333678}, {"X"=3585.196101527507, "Y"=3861.697172493809}, {"X"=3587.346185883872, "Y"=3863.779989812956}, {"X"=3589.5785361435096, "Y"=3863.850784101241}, {"X"=3591.811278765371, "Y"=3863.9078796131535}, {"X"=3594.044329687959, "Y"=3863.9512741990807}, {"X"=3596.2776048381675, "Y"=3863.9809662252396}, {"X"=3598.5232919465293, "Y"=3860.9969796734104}, {"X"=3600.734264958528, "Y"=3858.999249100845}, {"X"=3602.9124856990015, "Y"=3855.988086074595}, {"X"=3605.1110493698097, "Y"=3856.963411534487}, {"X"=3607.301239472894, "Y"=3856.9253309897736}, {"X"=3609.491154688439, "Y"=3856.8738124080837}, {"X"=3611.680712567374, "Y"=3856.8088577290628}, {"X"=3613.869830674083, "Y"=3856.730469398217}, {"X"=3616.0584265895063, "Y"=3856.6386503668236}, {"X"=3618.144197085594, "Y"=3854.5360180744956}, {"X"=3620.262010319799, "Y"=3853.4196527328386}, {"X"=3622.4301711150943, "Y"=3853.2886743496706}, {"X"=3624.5974874271237, "Y"=3853.1443948475926}, {"X"=3626.7638776576546, "Y"=3852.9868196586467}, {"X"=3628.847539169185, "Y"=3851.8192994761407}, {"X"=3631.0057187613443, "Y"=3851.6356714044987}, {"X"=3633.068785592103, "Y"=3850.4432270988605}, {"X"=3635.3184946920105, "Y"=3851.2287060202943}, {"X"=3637.3667730516813, "Y"=3850.01103449992}, {"X"=3639.513696966361, "Y"=3849.775167431953}, {"X"=3641.6591332126836, "Y"=3849.5261315266252}, {"X"=3643.803001016186, "Y"=3849.263936159999}, {"X"=3645.9452196614584, "Y"=3848.988591203581}, {"X"=3648.358922747992, "Y"=3850.681357632044}, {"X"=3650.5097527639764, "Y"=3850.3780313828506}, {"X"=3652.658681116318, "Y"=3850.06151359881}, {"X"=3654.805626899078, "Y"=3849.731816196638}, {"X"=3656.9505092809613, "Y"=3849.3889515892556}, {"X"=3659.093247508359, "Y"=3849.0329326853207}, {"X"=3661.233760908388, "Y"=3848.663772888745}, {"X"=3663.371968891928, "Y"=3848.2814860981853}, {"X"=3665.507790956657, "Y"=3847.8860867065237}, {"X"=3667.6411466900818, "Y"=3847.4775896003234}, {"X"=3669.771955772565, "Y"=3847.05601015927}, {"X"=3672.3063534491635, "Y"=3848.579677047995}, {"X"=3674.6529488935626, "Y"=3849.107343408149}, {"X"=3676.7936259622215, "Y"=3848.642709677937}, {"X"=3678.931411794267, "Y"=3848.1649497467597}, {"X"=3681.9745309554087, "Y"=3851.5695895191175}, {"X"=3682.265797573908, "Y"=3843.2802623943426}, {"X"=3684.3705770359, "Y"=3842.7690267959306}, {"X"=3685.982252627952, "Y"=3840.3058216266995}, {"X"=3689.072343340926, "Y"=3843.6438820228814}, {"X"=3690.408697130985, "Y"=3840.191515889326}, {"X"=3692.7571392126815, "Y"=3840.5952335618913}, {"X"=3694.845246150937, "Y"=3840.019674846277}, {"X"=3696.929782219281, "Y"=3839.4313145820856}, {"X"=3699.01066893611, "Y"=3838.830174920747}, {"X"=3701.0878279572144, "Y"=3838.2162784948305}, {"X"=3702.868939772559, "Y"=3836.6333038041093}, {"X"=3704.336338764959, "Y"=3834.086707926436}, {"X"=3706.9922024064654, "Y"=3835.3455958026198}, {"X"=3707.4988553411154, "Y"=3829.928774283708}, {"X"=3709.5212366069845, "Y"=3829.262962891481}, {"X"=3712.1823733908036, "Y"=3830.478615193792}, {"X"=3714.8625275878517, "Y"=3831.6739359011044}, {"X"=3716.8954783450504, "Y"=3830.9629090132034}, {"X"=3718.9240280535587, "Y"=3830.239421558839}, {"X"=3721.9818447869743, "Y"=3832.3197700143137}, {"X"=3725.069629579242, "Y"=3834.3749209449047}, {"X"=3726.0507345592364, "Y"=3830.79784206835}, {"X"=3728.078099090901, "Y"=3830.01818212526}, {"X"=3730.1006415545253, "Y"=3829.22609718414}, {"X"=3731.7450703059103, "Y"=3827.493872385562}, {"X"=3732.994252855881, "Y"=3824.8284604330506}, {"X"=3734.984859240635, "Y"=3824.006308234556}, {"X"=3737.750841547497, "Y"=3825.0133930362813}, {"X"=3741.3259774571916, "Y"=3827.8352758562896}, {"X"=3743.3348764721827, "Y"=3826.9619445542617}, {"X"=3745.338379010088, "Y"=3826.0763033198214}, {"X"=3747.3364096401688, "Y"=3825.17838549686}, {"X"=3749.747181353774, "Y"=3825.176539246914}, {"X"=3751.739608140834, "Y"=3824.2515864591355}, {"X"=3753.7263220174113, "Y"=3823.314425782394}, {"X"=3755.707248184851, "Y"=3822.3650925002603}, {"X"=3758.563218833701, "Y"=3823.19917331747}, {"X"=3760.989300513128, "Y"=3823.1152195739064}, {"X"=3762.5174303442213, "Y"=3821.229022403504}, {"X"=3764.9422991025817, "Y"=3821.11530322729}, {"X"=3766.909520570095, "Y"=3820.0971914013944}, {"X"=3770.273813595049, "Y"=3821.718554646446}, {"X"=3772.244636179431, "Y"=3820.6677179065823}, {"X"=3774.208973850614, "Y"=3819.604808208381}, {"X"=3775.1988034619967, "Y"=3816.779701473255}, {"X"=3776.1605593274253, "Y"=3813.95454661057}, {"X"=3778.083632037759, "Y"=3812.8677356331905}, {"X"=3781.0, "Y"=3813.5011961699665}]}]
  in  "merge threshold":dbl=40.0
  in  "split theshold":dbl=100.0
  in  "robotPos":cluster{"xPos":dbl, "yPos":dbl, "theta":dbl}={"xPos"=3600.0, "yPos"=3500.0, "theta"=90.0}
  out "odd line filter":cluster{"Line":cluster{"X":dbl, "Y":dbl}[]}[](graph)=[{"Line"=[{"X"=4045.262015510834, "Y"=-370.47254705975547}, {"X"=4021.5048604927456, "Y"=-373.1317628736815}, {"X"=3997.731836054895, "Y"=-375.64515746583857}, {"X"=3974.4237446268694, "Y"=-382.9895518092235}, {"X"=3948.973422153729, "Y"=-367.28671688954455}, {"X"=3924.2325152064327, "Y"=-357.3973448535103}, {"X"=3900.4802229985116, "Y"=-358.3172025621179}, {"X"=3876.8003772484603, "Y"=-360.08828281881506}, {"X"=3852.848497603733, "Y"=-357.72259724044125}, {"X"=3829.173196937117, "Y"=-359.2014259177531}, {"X"=3805.4892680291655, "Y"=-360.5349578426094}, {"X"=3782.314874586134, "Y"=-372.7109737888577}, {"X"=3758.6307242397825, "Y"=-375.7550610593494}, {"X"=3734.846552078191, "Y"=-376.65544089136483}, {"X"=3711.0000422297094, "Y"=-375.4106867047012}, {"X"=3687.3538586650116, "Y"=-382.0172981809769}, {"X"=3662.9108581038413, "Y"=-344.48530026226535}, {"X"=3639.320355486937, "Y"=-344.7989426814479}, {"X"=3615.7774597291873, "Y"=-356.96773019486045}, {"X"=3592.111253634981, "Y"=-356.9919325402784}, {"X"=3568.4453445476156, "Y"=-356.8709213194161}, {"X"=3543.4634903042615, "Y"=-448.5952721279782}, {"X"=3519.2364294721056, "Y"=-448.174039435899}]}, {"Line"=[{"X"=3206.375015694224, "Y"=-187.04805660711145}, {"X"=3183.7591240020847, "Y"=-184.5634114706845}, {"X"=3161.3956031641924, "Y"=-179.95410067521016}, {"X"=3138.8240858920867, "Y"=-177.1936005936277}, {"X"=3116.9225625935896, "Y"=-169.33743194447243}, {"X"=3094.5536322950015, "Y"=-165.31362496769452}, {"X"=3072.0732055742583, "Y"=-162.14326586595462}, {"X"=3050.50517501786, "Y"=-152.90178314690638}, {"X"=3029.3402803672284, "Y"=-141.5578375729042}, {"X"=3005.7198268817183, "Y"=-145.8835795782761}, {"X"=2983.360292949494, "Y"=-142.16851225868822}, {"X"=2961.369928605174, "Y"=-136.34646752894514}, {"X"=2939.069748166673, "Y"=-132.35945388277014}, {"X"=2916.0542503508345, "Y"=-132.16660019014535}, {"X"=2893.971646836575, "Y"=-126.92003834235948}, {"X"=2871.7305746338234, "Y"=-122.51965406356612}, {"X"=2849.516921363317, "Y"=-117.98288396725366}, {"X"=2827.3315233565468, "Y"=-113.3098988602519}, {"X"=2805.820540469126, "Y"=-105.57110400824695}, {"X"=2784.596507850818, "Y"=-96.72922875644326}, {"X"=2761.6344368770942, "Y"=-95.5538074919159}, {"X"=2738.656125118518, "Y"=-94.23186914869939}, {"X"=2716.6185475221346, "Y"=-88.87910208996846}, {"X"=2694.614228738148, "Y"=-83.39121576148591}, {"X"=2672.6439972167227, "Y"=-77.76841677907123}, {"X"=2650.708680124659, "Y"=-72.01091683792765}, {"X"=2628.809103314247, "Y"=-66.11893270467408}, {"X"=2606.946091292176, "Y"=-60.092686209182375}, {"X"=2584.5712899521213, "Y"=-55.85552783159346}, {"X"=2561.650151837172, "Y"=-53.3974718317445}, {"X"=2539.293725910705, "Y"=-48.87562477295114}, {"X"=2517.538201938755, "Y"=-42.30044684778477}, {"X"=2494.034809091436, "Y"=-41.3191040202214}, {"X"=2472.0225479250194, "Y"=-35.41905120318597}, {"X"=2450.0410633250167, "Y"=-29.382161789984366}, {"X"=2426.5130901879893, "Y"=-27.95301449719682}, {"X"=2404.2451890722396, "Y"=-22.58008172179325}, {"X"=2382.6535537697796, "Y"=-15.176756558716079}, {"X"=2359.4425731187703, "Y"=-12.355658331004179}, {"X"=2337.9145170954243, "Y"=-4.677621956337134}, {"X"=2315.0556519473794, "Y"=-0.6226620999336774}, {"X"=2293.6004238067435, "Y"=7.327506432634436}, {"X"=2270.057927743648, "Y"=9.802429024614412}, {"X"=2247.5821062096375, "Y"=15.231737897677704}, {"X"=2224.75536526262, "Y"=19.875548974426238}, {"X"=2200.815103181707, "Y"=21.88519100999474}, {"X"=2173.8166160981887, "Y"=16.65434452990621}, {"X"=2150.9317674680565, "Y"=21.778434678614303}, {"X"=2099.569445467065, "Y"=-40.16004596176299}, {"X"=1993.354962067471, "Y"=11.164560761459143}, {"X"=1971.9781148912214, "Y"=21.088425727543836}, {"X"=1946.7979336116412, "Y"=23.015253457493145}, {"X"=1925.494677341689, "Y"=33.224563893850245}, {"X"=1904.2544652507022, "Y"=43.564396465946174}, {"X"=1877.726652128255, "Y"=43.29368976613068}, {"X"=1842.55456574985, "Y"=26.26504384210375}, {"X"=1829.0405780564897, "Y"=52.23569166488596}, {"X"=1814.3917771697875, "Y"=75.5807390798177}, {"X"=1786.8645563340388, "Y"=74.22769832520271}, {"X"=1765.8785444190275, "Y"=85.41737745628188}, {"X"=1747.8331626322108, "Y"=102.00382481748511}, {"X"=1728.9542149611082, "Y"=116.9328013933573}, {"X"=1706.27398723018, "Y"=124.98862393636955}, {"X"=1685.60095559409, "Y"=136.67184194320134}, {"X"=1655.000000000001, "Y"=131.16117927853338}, {"X"=1628.3021546343343, "Y"=132.80359845458497}, {"X"=1607.6785425781395, "Y"=144.9650955174202}, {"X"=1587.1299402987506, "Y"=157.25290774813675}, {"X"=1566.6571214394316, "Y"=169.66657251754714}, {"X"=1546.2608567902394, "Y"=182.2056224581911}, {"X"=1525.9419142590123, "Y"=194.86958548192388}, {"X"=1494.9665691389255, "Y"=190.7828335152658}, {"X"=1455.735015665709, "Y"=174.34567686930814}, {"X"=1430.993243345882, "Y"=180.86838320792322}, {"X"=1410.668265549114, "Y"=194.23964018468632}, {"X"=1390.425714854734, "Y"=207.7353571705712}, {"X"=1357.3322111709276, "Y"=202.3364045208432}, {"X"=1334.8706766640394, "Y"=212.86551103190004}, {"X"=1311.3090852839077, "Y"=221.9063623965808}, {"X"=1275.0687472590512, "Y"=213.15186386282812}, {"X"=1254.9447924102292, "Y"=227.47924783415692}, {"X"=1234.9091275645433, "Y"=241.92984036216785}]}, {"Line"=[{"X"=270.96481001367874, "Y"=531.983035117094}, {"X"=568.1778192565093, "Y"=1887.4212377834735}, {"X"=558.3402951796288, "Y"=1906.0545053007447}, {"X"=548.617287871481, "Y"=1924.7477839649912}, {"X"=532.7695198753122, "Y"=1940.3275402206798}, {"X"=529.5162834990319, "Y"=1962.3115573360112}, {"X"=539.8702058904678, "Y"=1990.9109889727677}, {"X"=605.3325001870285, "Y"=2045.968512870534}, {"X"=601.8805011027116, "Y"=2066.9583152148466}, {"X"=605.8120277476805, "Y"=2091.3412809272986}, {"X"=674.3588639641607, "Y"=2145.452125934663}, {"X"=666.1025888247354, "Y"=2163.429021451132}, {"X"=657.9567732645942, "Y"=2181.4562381095116}, {"X"=619.7255133273352, "Y"=2186.221866490394}, {"X"=604.3804690989409, "Y"=2201.3512306693083}, {"X"=596.4685017416655, "Y"=2219.7564532597535}, {"X"=596.0480668191567, "Y"=2241.301551943805}, {"X"=707.6625662145384, "Y"=2308.879448114789}, {"X"=715.2401057472161, "Y"=2332.650715290977}, {"X"=717.4243259383866, "Y"=2354.0674176426273}, {"X"=719.7624075179106, "Y"=2375.413226623674}, {"X"=726.9221966011937, "Y"=2398.476992697342}, {"X"=720.2174633677091, "Y"=2416.1266025463633}, {"X"=715.4972516675775, "Y"=2434.5100212284015}, {"X"=731.5776225251552, "Y"=2460.4067793595614}, {"X"=730.9061825143826, "Y"=2480.0364386578276}, {"X"=719.9804701443845, "Y"=2496.014189517481}, {"X"=750.778902136793, "Y"=2526.316203538756}, {"X"=755.2887344326768, "Y"=2547.3102207148654}, {"X"=758.99836842379, "Y"=2567.9003650996783}, {"X"=769.5176591565032, "Y"=2590.550321252946}, {"X"=776.3916464972967, "Y"=2611.8356762232834}, {"X"=797.7559831999147, "Y"=2637.415238768894}, {"X"=794.4310781670474, "Y"=2655.202376397113}, {"X"=807.5266916718274, "Y"=2677.7994026548567}, {"X"=802.5343311689248, "Y"=2694.949174454491}, {"X"=797.6472936673199, "Y"=2712.1292559626913}, {"X"=792.8657631612118, "Y"=2729.3390003590985}, {"X"=738.9277025317801, "Y"=2733.377988406333}]}, {"Line"=[{"X"=914.1062820436955, "Y"=3224.364487333619}, {"X"=933.3686210466781, "Y"=3242.8656211598604}, {"X"=941.800605877364, "Y"=3260.131325333941}, {"X"=940.3788392110519, "Y"=3276.4462456507435}, {"X"=939.0572057782192, "Y"=3292.769582640043}, {"X"=948.8075824980851, "Y"=3309.887492835553}, {"X"=950.6845588015076, "Y"=3326.35469189397}, {"X"=952.6636881702325, "Y"=3342.7916921165966}, {"X"=952.7474978684022, "Y"=3359.091554695986}, {"X"=954.9294148586805, "Y"=3375.478517435108}, {"X"=960.2101388711521, "Y"=3391.956077999096}, {"X"=971.5896340437512, "Y"=3408.572716688413}, {"X"=974.0768960605492, "Y"=3424.7879517829642}, {"X"=981.6628112449193, "Y"=3441.081700787105}, {"X"=981.3505848148575, "Y"=3457.1486248702304}, {"X"=993.1363215681313, "Y"=3473.3398786074254}, {"X"=994.0218032440225, "Y"=3489.3398859076315}, {"X"=1020.0053964340373, "Y"=3505.2768902312037}, {"X"=1022.0862755609401, "Y"=3521.09097789895}, {"X"=1022.2642158658068, "Y"=3536.908362115882}, {"X"=1025.5385789953302, "Y"=3552.663001800286}, {"X"=1025.91017660836, "Y"=3568.4586087471434}, {"X"=1014.3851121986418, "Y"=3584.6442672599346}, {"X"=975.9825976478487, "Y"=3602.0229001404546}, {"X"=947.6873481122784, "Y"=3619.426113711875}, {"X"=927.497508824365, "Y"=3636.771468735349}, {"X"=928.3870318839645, "Y"=3653.1670610615342}, {"X"=905.4253651296312, "Y"=3671.0775763015645}, {"X"=1015.481200145904, "Y"=3743.8822937417594}, {"X"=1026.9761083045855, "Y"=3758.735488027024}, {"X"=1028.6121158613832, "Y"=3774.518395203543}, {"X"=1030.3449347186652, "Y"=3790.29096691764}, {"X"=1029.195583743087, "Y"=3806.4076587716963}, {"X"=1031.1240604595514, "Y"=3822.1760500878013}]}, {"Line"=[{"X"=-10.842185123417494, "Y"=3975.376392065428}, {"X"=-7.85735733306592, "Y"=3997.523154373408}, {"X"=-13.64461180448643, "Y"=4020.9353314725367}, {"X"=-10.380186862304981, "Y"=4043.0984315132105}, {"X"=-6.979833146683177, "Y"=4065.2410842048967}, {"X"=-1.4697297999809962, "Y"=4087.0407015995165}, {"X"=2.2000808792763564, "Y"=4109.12785355368}, {"X"=6.005346692003968, "Y"=4131.19207218844}, {"X"=10.929770378021203, "Y"=4153.0535099371555}, {"X"=16.96985273450491, "Y"=4174.693236802181}, {"X"=21.177142139041734, "Y"=4196.665595570732}, {"X"=25.51917220141786, "Y"=4218.611725273365}, {"X"=29.995779446655888, "Y"=4240.530799650704}, {"X"=34.606795333023456, "Y"=4262.421993461985}, {"X"=39.35204625837832, "Y"=4284.2844825161355}, {"X"=44.23135356670491, "Y"=4306.117443702798}, {"X"=50.2184105341189, "Y"=4327.69297876029}, {"X"=54.39139747939407, "Y"=4349.6914956217215}, {"X"=60.64276863692294, "Y"=4371.191935682311}, {"X"=66.05492926119678, "Y"=4392.892623444115}, {"X"=71.60014091999074, "Y"=4414.559694303313}, {"X"=76.31174166907931, "Y"=4436.449175396509}, {"X"=78.26458215041703, "Y"=4459.103564097132}, {"X"=80.36291249774058, "Y"=4481.769205199782}, {"X"=86.453191266457, "Y"=4503.346810847743}, {"X"=92.675753086658, "Y"=4524.88664105537}, {"X"=99.03036368240737, "Y"=4546.387884860228}, {"X"=96.90968228848942, "Y"=4570.479904508192}, {"X"=101.63490128460626, "Y"=4592.550518781641}, {"X"=108.40452097556545, "Y"=4613.995516533227}, {"X"=117.20720403105815, "Y"=4634.778983038918}, {"X"=124.23563956341286, "Y"=4656.127635998224}]}, {"Line"=[{"X"=116.24405358750664, "Y"=4682.575792850332}, {"X"=1470.8259571533572, "Y"=4356.529564736725}, {"X"=1476.1216048608221, "Y"=4369.577807134607}, {"X"=1493.49744902776, "Y"=4377.593871188402}, {"X"=1498.9219181053986, "Y"=4390.502607397701}, {"X"=1938.6303433573366, "Y"=4228.317831710194}, {"X"=1943.130492374914, "Y"=4238.4980939056}, {"X"=2064.2835911828975, "Y"=4195.824052250209}, {"X"=2157.596803563967, "Y"=4164.241687122327}, {"X"=2184.342933978691, "Y"=4162.483261240568}, {"X"=2240.815053624293, "Y"=4146.251716860904}, {"X"=2273.6207227573095, "Y"=4140.661387084596}, {"X"=2307.20330673012, "Y"=4134.252875334802}, {"X"=2353.1869782092754, "Y"=4121.213561259799}, {"X"=2382.006623386713, "Y"=4116.211923388506}, {"X"=2411.6065232364003, "Y"=4110.423577842243}, {"X"=2447.295432626557, "Y"=4101.059215349373}, {"X"=2473.9850587374376, "Y"=4095.9583475826716}, {"X"=2498.805913782341, "Y"=4091.4994374293647}, {"X"=2516.504578766092, "Y"=4090.5875651968613}, {"X"=2551.6517061741442, "Y"=4079.8015650482653}, {"X"=2575.2872437016113, "Y"=4074.968492249235}, {"X"=2594.4778607566627, "Y"=4072.3410062991315}, {"X"=2611.865014281955, "Y"=4070.5}, {"X"=2636.9576668055656, "Y"=4063.91973229833}, {"X"=2659.3520795735667, "Y"=4058.5852574114597}, {"X"=2678.2173574415674, "Y"=4055.061041578305}, {"X"=2691.0289338111706, "Y"=4054.9744145738096}, {"X"=2721.660278831192, "Y"=4043.6987531870027}, {"X"=2739.4124804842736, "Y"=4040.041777322615}, {"X"=2750.3361329295954, "Y"=4040.4815565724384}, {"X"=2767.115634515412, "Y"=4037.014556349579}, {"X"=2782.982986635797, "Y"=4033.9093554840906}, {"X"=2807.9514900820814, "Y"=4024.5561532732263}, {"X"=2814.50634246743, "Y"=4027.177118221292}, {"X"=2830.9861725688024, "Y"=4022.9892285885253}, {"X"=2853.1485517299434, "Y"=4014.6473688040373}, {"X"=2857.1403612634576, "Y"=4018.6478160912407}, {"X"=2872.582789543413, "Y"=4014.533965770538}, {"X"=2885.50776424397, "Y"=4011.997895546798}, {"X"=2893.5183185882197, "Y"=4012.847573680118}, {"X"=2899.900941786414, "Y"=4014.8031747070427}, {"X"=2912.6967434174403, "Y"=4011.9211203798964}, {"X"=2931.0186065410116, "Y"=4004.685937198244}, {"X"=2945.2522496038464, "Y"=4000.2813042191124}, {"X"=2954.661095425663, "Y"=3999.3933301945417}, {"X"=2967.182500916552, "Y"=3995.94154177057}, {"X"=2976.503747613994, "Y"=3994.8418164025816}, {"X"=2988.905267857863, "Y"=3991.1407418939402}, {"X"=2993.4815525575614, "Y"=3993.618651300793}, {"X"=3003.4671589723284, "Y"=3991.6071292968145}, {"X"=3015.7083674570613, "Y"=3987.569777714234}, {"X"=3022.5302826587013, "Y"=3987.918769421469}, {"X"=3030.0942129466903, "Y"=3987.552452442963}, {"X"=3046.702190705782, "Y"=3979.2551869622475}, {"X"=3057.1716590001784, "Y"=3976.0476785022497}, {"X"=3067.5806510774983, "Y"=3972.729983069553}, {"X"=3074.953442415055, "Y"=3971.9768133798516}, {"X"=3079.338473615689, "Y"=3973.843407618128}, {"X"=3090.3454777343677, "Y"=3969.5756253620816}, {"X"=3094.698855111437, "Y"=3971.3297709399512}, {"X"=3103.4168856555025, "Y"=3968.92879048734}, {"X"=3107.7491971523373, "Y"=3970.584898924553}, {"X"=3123.58038741206, "Y"=3961.0784670113726}, {"X"=3127.132781099316, "Y"=3963.2932044495506}, {"X"=3141.3442900960695, "Y"=3954.9186078547696}, {"X"=3145.5555703671926, "Y"=3956.307199565942}, {"X"=3151.8704643852734, "Y"=3955.5226880296186}, {"X"=3156.0677567657553, "Y"=3956.8294686390223}, {"X"=3159.5716639723732, "Y"=3958.823365603732}, {"X"=3175.4683402686765, "Y"=3947.7296839453106}, {"X"=3178.2235496518883, "Y"=3950.3261328545645}, {"X"=3180.994638680067, "Y"=3952.9056272394423}, {"X"=3195.249435679037, "Y"=3942.9187066289505}, {"X"=3197.974753086856, "Y"=3945.3938715838212}, {"X"=3201.380681173798, "Y"=3947.1058472649793}, {"X"=3206.7751036892987, "Y"=3946.541354099974}, {"X"=3212.803756375196, "Y"=3945.173077491038}, {"X"=3218.8006896511197, "Y"=3943.7477727150167}, {"X"=3224.1184753772477, "Y"=3943.0283054696115}, {"X"=3228.7707174038055, "Y"=3943.026883770178}, {"X"=3236.596467994627, "Y"=3939.1330924970466}, {"X"=3243.09464444919, "Y"=3936.7087899036956}, {"X"=3247.0370537459103, "Y"=3937.33414978896}, {"X"=3255.336482079424, "Y"=3932.453534399492}, {"X"=3258.6149065322234, "Y"=3933.7743860095907}, {"X"=3264.351012075589, "Y"=3931.9129043051607}, {"X"=3269.4425440482646, "Y"=3930.7908637781406}, {"X"=3272.6959317916744, "Y"=3932.0139429859637}, {"X"=3277.1498206927595, "Y"=3931.6118183290196}, {"X"=3284.5566606113143, "Y"=3927.1492709057507}, {"X"=3290.7181866922274, "Y"=3924.2284289826134}, {"X"=3293.3270255400894, "Y"=3926.118160532863}, {"X"=3297.105706031337, "Y"=3926.3614038362584}, {"X"=3304.8947253046604, "Y"=3920.8430548874344}, {"X"=3308.6207253100038, "Y"=3921.001328122765}, {"X"=3311.2094260290082, "Y"=3922.7812725103904}, {"X"=3314.926933145405, "Y"=3922.8869193461956}, {"X"=3318.0809533830084, "Y"=3923.7955298897887}, {"X"=3324.527865814621, "Y"=3919.6654659217893}, {"X"=3329.8261174974987, "Y"=3917.1511395328134}, {"X"=3334.0061420335082, "Y"=3916.2730684587964}, {"X"=3338.165158372983, "Y"=3915.359501769437}, {"X"=3341.2467531813195, "Y"=3916.109068948024}, {"X"=3349.556141722818, "Y"=3908.312225938973}, {"X"=3352.0662129768757, "Y"=3909.8412342021875}, {"X"=3356.12266085134, "Y"=3908.7784772340265}, {"X"=3358.635469356694, "Y"=3910.2671853162724}, {"X"=3361.659135341594, "Y"=3910.875446131651}, {"X"=3366.6669726322425, "Y"=3907.989826269476}, {"X"=3370.1569787062945, "Y"=3907.671663919117}, {"X"=3375.5773121030506, "Y"=3903.8297378315624}, {"X"=3379.9809532133554, "Y"=3901.6909496753647}, {"X"=3381.0248231909495, "Y"=3905.6733562134013}, {"X"=3384.9268861109003, "Y"=3904.360675241852}, {"X"=3387.4120452614275, "Y"=3905.672727084371}, {"X"=3391.740097239402, "Y"=3903.415186751994}, {"X"=3396.9388950941193, "Y"=3899.337185439076}, {"X"=3399.3930045680063, "Y"=3900.5756275458457}, {"X"=3402.2969554721067, "Y"=3900.902115465112}, {"X"=3404.7605663121444, "Y"=3902.107651672093}, {"X"=3407.231527806511, "Y"=3903.2980487532614}, {"X"=3410.1354521890526, "Y"=3903.5684000074143}, {"X"=3415.9764364638286, "Y"=3897.4661344862584}, {"X"=3419.2478453327217, "Y"=3896.7677640423126}, {"X"=3421.685769173619, "Y"=3897.8693693724063}, {"X"=3424.1304064445235, "Y"=3898.9559951456195}, {"X"=3428.570407478858, "Y"=3895.4401279688686}, {"X"=3431.000009603355, "Y"=3896.484556125373}, {"X"=3434.595352849846, "Y"=3894.747137673135}, {"X"=3437.0205894479313, "Y"=3895.754610505172}, {"X"=3440.2021866047417, "Y"=3894.893224598871}, {"X"=3442.997631366253, "Y"=3894.937028199931}, {"X"=3445.7875834697406, "Y"=3894.9614292407523}, {"X"=3447.855938217865, "Y"=3896.8339507456913}, {"X"=3453.1117300168457, "Y"=3890.272771457805}, {"X"=3455.509163854388, "Y"=3891.166714164104}, {"X"=3457.912037690245, "Y"=3892.0459296647036}, {"X"=3460.9901878630535, "Y"=3891.0259225801415}, {"X"=3465.367148692672, "Y"=3886.2058976101466}, {"X"=3467.7393979566095, "Y"=3887.0247190388745}, {"X"=3470.7517532769834, "Y"=3885.9324950286336}, {"X"=3473.433962618886, "Y"=3885.7681145217193}, {"X"=3475.497470820703, "Y"=3887.489509829567}, {"X"=3479.0776275398593, "Y"=3884.430461642429}, {"X"=3482.0271182627307, "Y"=3883.2537007970104}, {"X"=3483.804285900354, "Y"=3885.8854182589353}, {"X"=3486.7391138662306, "Y"=3884.672551233115}, {"X"=3490.4843260336584, "Y"=3880.555274770562}, {"X"=3492.821430903891, "Y"=3881.2200864677916}, {"X"=3494.6330890219583, "Y"=3883.7991845626375}, {"X"=3497.507658139402, "Y"=3882.506627210471}, {"X"=3499.8566040708733, "Y"=3883.1283078183887}, {"X"=3502.9501588268386, "Y"=3880.828476257047}, {"X"=3505.2887053640984, "Y"=3881.4167938992614}, {"X"=3507.6308177280707, "Y"=3881.9907514147626}, {"X"=3510.434543069118, "Y"=3880.603506190842}, {"X"=3513.2177495607757, "Y"=3879.196309328959}, {"X"=3516.631613886397, "Y"=3874.8409158520626}, {"X"=3518.9331638941576, "Y"=3875.3453983783315}, {"X"=3521.6479859911105, "Y"=3873.8782715012344}, {"X"=3524.1426355863878, "Y"=3873.3720132310673}, {"X"=3526.241947276591, "Y"=3874.81161889468}, {"X"=3528.54313660979, "Y"=3875.257134075334}, {"X"=3530.847016253508, "Y"=3875.6885210369855}, {"X"=3532.2785452725334, "Y"=3881.0286138462516}, {"X"=3534.6177677323685, "Y"=3881.4369721247554}, {"X"=3537.448138216478, "Y"=3878.8710395205935}, {"X"=3540.244540164776, "Y"=3876.284845588925}, {"X"=3542.554505452179, "Y"=3876.644414741751}, {"X"=3545.879582520246, "Y"=3870.0634815971675}, {"X"=3548.2899011305954, "Y"=3869.3982480669288}, {"X"=3550.5574595983317, "Y"=3869.7085814511606}, {"X"=3552.953349041593, "Y"=3869.013025018898}, {"X"=3555.459217026101, "Y"=3867.3092956243718}, {"X"=3557.713822962267, "Y"=3867.5756782371946}, {"X"=3560.1863992142376, "Y"=3865.839961174927}, {"X"=3562.4319004958415, "Y"=3866.0773660029336}, {"X"=3564.486853239697, "Y"=3868.291754465371}, {"X"=3566.657445372384, "Y"=3869.498679362869}, {"X"=3568.9252743111374, "Y"=3869.696309723754}, {"X"=3571.1942731957497, "Y"=3869.880021227531}, {"X"=3573.4643565996953, "Y"=3870.049806957566}, {"X"=3575.9970515725377, "Y"=3866.2142248285672}, {"X"=3578.4223891140427, "Y"=3863.359885937419}, {"X"=3580.7586355337407, "Y"=3861.4882707550505}, {"X"=3582.9770480783645, "Y"=3861.5995286333678}, {"X"=3585.196101527507, "Y"=3861.697172493809}, {"X"=3587.346185883872, "Y"=3863.779989812956}, {"X"=3589.5785361435096, "Y"=3863.850784101241}, {"X"=3591.811278765371, "Y"=3863.9078796131535}, {"X"=3594.044329687959, "Y"=3863.9512741990807}, {"X"=3596.2776048381675, "Y"=3863.9809662252396}, {"X"=3598.5232919465293, "Y"=3860.9969796734104}, {"X"=3600.734264958528, "Y"=3858.999249100845}, {"X"=3602.9124856990015, "Y"=3855.988086074595}, {"X"=3605.1110493698097, "Y"=3856.963411534487}, {"X"=3607.301239472894, "Y"=3856.9253309897736}, {"X"=3609.491154688439, "Y"=3856.8738124080837}, {"X"=3611.680712567374, "Y"=3856.8088577290628}, {"X"=3613.869830674083, "Y"=3856.730469398217}, {"X"=3616.0584265895063, "Y"=3856.6386503668236}, {"X"=3618.144197085594, "Y"=3854.5360180744956}, {"X"=3620.262010319799, "Y"=3853.4196527328386}, {"X"=3622.4301711150943, "Y"=3853.2886743496706}, {"X"=3624.5974874271237, "Y"=3853.1443948475926}, {"X"=3626.7638776576546, "Y"=3852.9868196586467}, {"X"=3628.847539169185, "Y"=3851.8192994761407}, {"X"=3631.0057187613443, "Y"=3851.6356714044987}, {"X"=3633.068785592103, "Y"=3850.4432270988605}, {"X"=3635.3184946920105, "Y"=3851.2287060202943}, {"X"=3637.3667730516813, "Y"=3850.01103449992}, {"X"=3639.513696966361, "Y"=3849.775167431953}, {"X"=3641.6591332126836, "Y"=3849.5261315266252}, {"X"=3643.803001016186, "Y"=3849.263936159999}, {"X"=3645.9452196614584, "Y"=3848.988591203581}, {"X"=3648.358922747992, "Y"=3850.681357632044}, {"X"=3650.5097527639764, "Y"=3850.3780313828506}, {"X"=3652.658681116318, "Y"=3850.06151359881}, {"X"=3654.805626899078, "Y"=3849.731816196638}, {"X"=3656.9505092809613, "Y"=3849.3889515892556}, {"X"=3659.093247508359, "Y"=3849.0329326853207}, {"X"=3661.233760908388, "Y"=3848.663772888745}, {"X"=3663.371968891928, "Y"=3848.2814860981853}, {"X"=3665.507790956657, "Y"=3847.8860867065237}, {"X"=3667.6411466900818, "Y"=3847.4775896003234}, {"X"=3669.771955772565, "Y"=3847.05601015927}, {"X"=3672.3063534491635, "Y"=3848.579677047995}, {"X"=3674.6529488935626, "Y"=3849.107343408149}, {"X"=3676.7936259622215, "Y"=3848.642709677937}, {"X"=3678.931411794267, "Y"=3848.1649497467597}, {"X"=3681.9745309554087, "Y"=3851.5695895191175}, {"X"=3682.265797573908, "Y"=3843.2802623943426}, {"X"=3684.3705770359, "Y"=3842.7690267959306}, {"X"=3685.982252627952, "Y"=3840.3058216266995}, {"X"=3689.072343340926, "Y"=3843.6438820228814}, {"X"=3690.408697130985, "Y"=3840.191515889326}, {"X"=3692.7571392126815, "Y"=3840.5952335618913}, {"X"=3694.845246150937, "Y"=3840.019674846277}, {"X"=3696.929782219281, "Y"=3839.4313145820856}, {"X"=3699.01066893611, "Y"=3838.830174920747}, {"X"=3701.0878279572144, "Y"=3838.2162784948305}, {"X"=3702.868939772559, "Y"=3836.6333038041093}, {"X"=3704.336338764959, "Y"=3834.086707926436}, {"X"=3706.9922024064654, "Y"=3835.3455958026198}, {"X"=3707.4988553411154, "Y"=3829.928774283708}, {"X"=3709.5212366069845, "Y"=3829.262962891481}, {"X"=3712.1823733908036, "Y"=3830.478615193792}, {"X"=3714.8625275878517, "Y"=3831.6739359011044}, {"X"=3716.8954783450504, "Y"=3830.9629090132034}, {"X"=3718.9240280535587, "Y"=3830.239421558839}, {"X"=3721.9818447869743, "Y"=3832.3197700143137}, {"X"=3725.069629579242, "Y"=3834.3749209449047}, {"X"=3726.0507345592364, "Y"=3830.79784206835}, {"X"=3728.078099090901, "Y"=3830.01818212526}, {"X"=3730.1006415545253, "Y"=3829.22609718414}, {"X"=3731.7450703059103, "Y"=3827.493872385562}, {"X"=3732.994252855881, "Y"=3824.8284604330506}, {"X"=3734.984859240635, "Y"=3824.006308234556}, {"X"=3737.750841547497, "Y"=3825.0133930362813}, {"X"=3741.3259774571916, "Y"=3827.8352758562896}, {"X"=3743.3348764721827, "Y"=3826.9619445542617}, {"X"=3745.338379010088, "Y"=3826.0763033198214}, {"X"=3747.3364096401688, "Y"=3825.17838549686}, {"X"=3749.747181353774, "Y"=3825.176539246914}, {"X"=3751.739608140834, "Y"=3824.2515864591355}, {"X"=3753.7263220174113, "Y"=3823.314425782394}, {"X"=3755.707248184851, "Y"=3822.3650925002603}, {"X"=3758.563218833701, "Y"=3823.19917331747}, {"X"=3760.989300513128, "Y"=3823.1152195739064}, {"X"=3762.5174303442213, "Y"=3821.229022403504}, {"X"=3764.9422991025817, "Y"=3821.11530322729}, {"X"=3766.909520570095, "Y"=3820.0971914013944}, {"X"=3770.273813595049, "Y"=3821.718554646446}, {"X"=3772.244636179431, "Y"=3820.6677179065823}, {"X"=3774.208973850614, "Y"=3819.604808208381}, {"X"=3775.1988034619967, "Y"=3816.779701473255}, {"X"=3776.1605593274253, "Y"=3813.95454661057}, {"X"=3778.083632037759, "Y"=3812.8677356331905}, {"X"=3781.0, "Y"=3813.5011961699665}]}]
  out "Raw Lidar Data":cluster{"Line":cluster{"X":dbl, "Y":dbl}[]}[](graph)=[{"Line"=[{"X"=4702.197140342376, "Y"=1516.6890148488842}, {"X"=4604.143011328081, "Y"=1554.8990224667068}, {"X"=4592.189193390564, "Y"=1548.7743327541575}, {"X"=4594.527091192987, "Y"=1514.1105607604393}, {"X"=4582.323180976402, "Y"=1508.045641055899}, {"X"=4580.564941005001, "Y"=1480.4660447341178}, {"X"=4571.173600402096, "Y"=1468.1717991222706}, {"X"=4570.608002262242, "Y"=1436.9149057916925}, {"X"=4568.854651859388, "Y"=1407.4043239148123}, {"X"=4555.996487758588, "Y"=1401.4989360514387}, {"X"=4548.828017241294, "Y"=1382.8969336147202}, {"X"=4541.87041502761, "Y"=1363.3893379242631}, {"X"=4537.493154460165, "Y"=1337.4654718732627}, {"X"=4530.088114201489, "Y"=1317.9550646650014}, {"X"=4520.932883548637, "Y"=1302.1438573012124}, {"X"=4510.476099602794, "Y"=1289.1372109395656}, {"X"=4513.398299571488, "Y"=1242.805159863262}, {"X"=4500.178610642434, "Y"=1194.5058080875897}, {"X"=4045.262015510834, "Y"=-370.47254705975547}, {"X"=4021.5048604927456, "Y"=-373.1317628736815}, {"X"=3997.731836054895, "Y"=-375.64515746583857}, {"X"=3974.4237446268694, "Y"=-382.9895518092235}, {"X"=3948.973422153729, "Y"=-367.28671688954455}, {"X"=3924.2325152064327, "Y"=-357.3973448535103}, {"X"=3900.4802229985116, "Y"=-358.3172025621179}, {"X"=3876.8003772484603, "Y"=-360.08828281881506}, {"X"=3852.848497603733, "Y"=-357.72259724044125}, {"X"=3829.173196937117, "Y"=-359.2014259177531}, {"X"=3805.4892680291655, "Y"=-360.5349578426094}, {"X"=3782.314874586134, "Y"=-372.7109737888577}, {"X"=3758.6307242397825, "Y"=-375.7550610593494}, {"X"=3734.846552078191, "Y"=-376.65544089136483}, {"X"=3711.0000422297094, "Y"=-375.4106867047012}, {"X"=3687.3538586650116, "Y"=-382.0172981809769}, {"X"=3662.9108581038413, "Y"=-344.48530026226535}, {"X"=3639.320355486937, "Y"=-344.7989426814479}, {"X"=3615.7774597291873, "Y"=-356.96773019486045}, {"X"=3592.111253634981, "Y"=-356.9919325402784}, {"X"=3568.4453445476156, "Y"=-356.8709213194161}, {"X"=3543.4634903042615, "Y"=-448.5952721279782}, {"X"=3519.2364294721056, "Y"=-448.174039435899}, {"X"=3495.0124093427307, "Y"=-447.6041602227524}, {"X"=3447.5484157840283, "Y"=-421.03742834342756}, {"X"=3429.4298217719656, "Y"=-288.161798854328}, {"X"=3406.547081777543, "Y"=-280.0530377801865}, {"X"=3383.3567540665535, "Y"=-278.7948745587423}, {"X"=3360.744841438998, "Y"=-268.4125263964861}, {"X"=3337.6268007773465, "Y"=-266.8735450409895}, {"X"=3312.0237005706044, "Y"=-298.09829401069464}, {"X"=3288.724428624859, "Y"=-296.2598065286679}, {"X"=3270.706969868897, "Y"=-234.51028922227988}, {"X"=3249.771498047274, "Y"=-211.51235972884115}, {"X"=3227.8050984298025, "Y"=-201.33367250848505}, {"X"=3206.375015694224, "Y"=-187.04805660711145}, {"X"=3183.7591240020847, "Y"=-184.5634114706845}, {"X"=3161.3956031641924, "Y"=-179.95410067521016}, {"X"=3138.8240858920867, "Y"=-177.1936005936277}, {"X"=3116.9225625935896, "Y"=-169.33743194447243}, {"X"=3094.5536322950015, "Y"=-165.31362496769452}, {"X"=3072.0732055742583, "Y"=-162.14326586595462}, {"X"=3050.50517501786, "Y"=-152.90178314690638}, {"X"=3029.3402803672284, "Y"=-141.5578375729042}, {"X"=3005.7198268817183, "Y"=-145.8835795782761}, {"X"=2983.360292949494, "Y"=-142.16851225868822}, {"X"=2961.369928605174, "Y"=-136.34646752894514}, {"X"=2939.069748166673, "Y"=-132.35945388277014}, {"X"=2916.0542503508345, "Y"=-132.16660019014535}, {"X"=2893.971646836575, "Y"=-126.92003834235948}, {"X"=2871.7305746338234, "Y"=-122.51965406356612}, {"X"=2849.516921363317, "Y"=-117.98288396725366}, {"X"=2827.3315233565468, "Y"=-113.3098988602519}, {"X"=2805.820540469126, "Y"=-105.57110400824695}, {"X"=2784.596507850818, "Y"=-96.72922875644326}, {"X"=2761.6344368770942, "Y"=-95.5538074919159}, {"X"=2738.656125118518, "Y"=-94.23186914869939}, {"X"=2716.6185475221346, "Y"=-88.87910208996846}, {"X"=2694.614228738148, "Y"=-83.39121576148591}, {"X"=2672.6439972167227, "Y"=-77.76841677907123}, {"X"=2650.708680124659, "Y"=-72.01091683792765}, {"X"=2628.809103314247, "Y"=-66.11893270467408}, {"X"=2606.946091292176, "Y"=-60.092686209182375}, {"X"=2584.5712899521213, "Y"=-55.85552783159346}, {"X"=2561.650151837172, "Y"=-53.3974718317445}, {"X"=2539.293725910705, "Y"=-48.87562477295114}, {"X"=2517.538201938755, "Y"=-42.30044684778477}, {"X"=2494.034809091436, "Y"=-41.3191040202214}, {"X"=2472.0225479250194, "Y"=-35.41905120318597}, {"X"=2450.0410633250167, "Y"=-29.382161789984366}, {"X"=2426.5130901879893, "Y"=-27.95301449719682}, {"X"=2404.2451890722396, "Y"=-22.58008172179325}, {"X"=2382.6535537697796, "Y"=-15.176756558716079}, {"X"=2359.4425731187703, "Y"=-12.355658331004179}, {"X"=2337.9145170954243, "Y"=-4.677621956337134}, {"X"=2315.0556519473794, "Y"=-0.6226620999336774}, {"X"=2293.6004238067435, "Y"=7.327506432634436}, {"X"=2270.057927743648, "Y"=9.802429024614412}, {"X"=2247.5821062096375, "Y"=15.231737897677704}, {"X"=2224.75536526262, "Y"=19.875548974426238}, {"X"=2200.815103181707, "Y"=21.88519100999474}, {"X"=2173.8166160981887, "Y"=16.65434452990621}, {"X"=2150.9317674680565, "Y"=21.778434678614303}, {"X"=2099.569445467065, "Y"=-40.16004596176299}, {"X"=1993.354962067471, "Y"=11.164560761459143}, {"X"=1971.9781148912214, "Y"=21.088425727543836}, {"X"=1946.7979336116412, "Y"=23.015253457493145}, {"X"=1925.494677341689, "Y"=33.224563893850245}, {"X"=1904.2544652507022, "Y"=43.564396465946174}, {"X"=1877.726652128255, "Y"=43.29368976613068}, {"X"=1842.55456574985, "Y"=26.26504384210375}, {"X"=1829.0405780564897, "Y"=52.23569166488596}, {"X"=1814.3917771697875, "Y"=75.5807390798177}, {"X"=1786.8645563340388, "Y"=74.22769832520271}, {"X"=1765.8785444190275, "Y"=85.41737745628188}, {"X"=1747.8331626322108, "Y"=102.00382481748511}, {"X"=1728.9542149611082, "Y"=116.9328013933573}, {"X"=1706.27398723018, "Y"=124.98862393636955}, {"X"=1685.60095559409, "Y"=136.67184194320134}, {"X"=1655.000000000001, "Y"=131.16117927853338}, {"X"=1628.3021546343343, "Y"=132.80359845458497}, {"X"=1607.6785425781395, "Y"=144.9650955174202}, {"X"=1587.1299402987506, "Y"=157.25290774813675}, {"X"=1566.6571214394316, "Y"=169.66657251754714}, {"X"=1546.2608567902394, "Y"=182.2056224581911}, {"X"=1525.9419142590123, "Y"=194.86958548192388}, {"X"=1494.9665691389255, "Y"=190.7828335152658}, {"X"=1455.735015665709, "Y"=174.34567686930814}, {"X"=1430.993243345882, "Y"=180.86838320792322}, {"X"=1410.668265549114, "Y"=194.23964018468632}, {"X"=1390.425714854734, "Y"=207.7353571705712}, {"X"=1357.3322111709276, "Y"=202.3364045208432}, {"X"=1334.8706766640394, "Y"=212.86551103190004}, {"X"=1311.3090852839077, "Y"=221.9063623965808}, {"X"=1275.0687472590512, "Y"=213.15186386282812}, {"X"=1254.9447924102292, "Y"=227.47924783415692}, {"X"=1234.9091275645433, "Y"=241.92984036216785}, {"X"=713.0611631530592, "Y"=-278.30771011372644}, {"X"=573.1977201747654, "Y"=410.6484565778592}, {"X"=592.3260462109588, "Y"=467.61836377757436}, {"X"=573.776320891091, "Y"=486.13018794763866}, {"X"=516.8456561375579, "Y"=466.8853810114342}, {"X"=481.7982266209283, "Y"=469.8314072488288}, {"X"=435.128765874887, "Y"=462.0139777465424}, {"X"=416.5476118831816, "Y"=481.49045179689256}, {"X"=381.2994394025459, "Y"=485.35794807913635}, {"X"=362.86253464191304, "Y"=505.1642732238183}, {"X"=342.3329127440702, "Y"=523.0595994193186}, {"X"=336.7475675292044, "Y"=554.4950242830287}, {"X"=270.96481001367874, "Y"=531.983035117094}, {"X"=568.1778192565093, "Y"=1887.4212377834735}, {"X"=558.3402951796288, "Y"=1906.0545053007447}, {"X"=548.617287871481, "Y"=1924.7477839649912}, {"X"=532.7695198753122, "Y"=1940.3275402206798}, {"X"=529.5162834990319, "Y"=1962.3115573360112}, {"X"=539.8702058904678, "Y"=1990.9109889727677}, {"X"=605.3325001870285, "Y"=2045.968512870534}, {"X"=601.8805011027116, "Y"=2066.9583152148466}, {"X"=605.8120277476805, "Y"=2091.3412809272986}, {"X"=674.3588639641607, "Y"=2145.452125934663}, {"X"=666.1025888247354, "Y"=2163.429021451132}, {"X"=657.9567732645942, "Y"=2181.4562381095116}, {"X"=619.7255133273352, "Y"=2186.221866490394}, {"X"=604.3804690989409, "Y"=2201.3512306693083}, {"X"=596.4685017416655, "Y"=2219.7564532597535}, {"X"=596.0480668191567, "Y"=2241.301551943805}, {"X"=707.6625662145384, "Y"=2308.879448114789}, {"X"=715.2401057472161, "Y"=2332.650715290977}, {"X"=717.4243259383866, "Y"=2354.0674176426273}, {"X"=719.7624075179106, "Y"=2375.413226623674}, {"X"=726.9221966011937, "Y"=2398.476992697342}, {"X"=720.2174633677091, "Y"=2416.1266025463633}, {"X"=715.4972516675775, "Y"=2434.5100212284015}, {"X"=731.5776225251552, "Y"=2460.4067793595614}, {"X"=730.9061825143826, "Y"=2480.0364386578276}, {"X"=719.9804701443845, "Y"=2496.014189517481}, {"X"=750.778902136793, "Y"=2526.316203538756}, {"X"=755.2887344326768, "Y"=2547.3102207148654}, {"X"=758.99836842379, "Y"=2567.9003650996783}, {"X"=769.5176591565032, "Y"=2590.550321252946}, {"X"=776.3916464972967, "Y"=2611.8356762232834}, {"X"=797.7559831999147, "Y"=2637.415238768894}, {"X"=794.4310781670474, "Y"=2655.202376397113}, {"X"=807.5266916718274, "Y"=2677.7994026548567}, {"X"=802.5343311689248, "Y"=2694.949174454491}, {"X"=797.6472936673199, "Y"=2712.1292559626913}, {"X"=792.8657631612118, "Y"=2729.3390003590985}, {"X"=738.9277025317801, "Y"=2733.377988406333}, {"X"=734.2776571765958, "Y"=2750.94762943921}, {"X"=804.3507531766409, "Y"=2787.56032624791}, {"X"=811.678247143569, "Y"=2807.6194669492497}, {"X"=814.2862759422133, "Y"=2826.386574067813}, {"X"=836.487585483886, "Y"=2849.676899675769}, {"X"=853.0200522133496, "Y"=2871.330638206337}, {"X"=849.2143206481433, "Y"=2888.19762482257}, {"X"=849.4220025087889, "Y"=2905.932091661871}, {"X"=845.8286492029479, "Y"=2922.82050413347}, {"X"=842.3389888918005, "Y"=2939.7306470868652}, {"X"=844.8402464495775, "Y"=2957.8203873106486}, {"X"=851.3888451759594, "Y"=2976.606534644484}, {"X"=857.0804053085021, "Y"=2995.110807149304}, {"X"=861.9106586397288, "Y"=3013.350476493323}, {"X"=892.4874355899142, "Y"=3035.904413335442}, {"X"=1025.8475465905508, "Y"=3075.0057099135174}, {"X"=1023.2882883425077, "Y"=3090.8084128343826}, {"X"=1304.545062912477, "Y"=3149.899111968396}, {"X"=1302.4400955384413, "Y"=3163.990349229975}, {"X"=914.1062820436955, "Y"=3224.364487333619}, {"X"=933.3686210466781, "Y"=3242.8656211598604}, {"X"=941.800605877364, "Y"=3260.131325333941}, {"X"=940.3788392110519, "Y"=3276.4462456507435}, {"X"=939.0572057782192, "Y"=3292.769582640043}, {"X"=948.8075824980851, "Y"=3309.887492835553}, {"X"=950.6845588015076, "Y"=3326.35469189397}, {"X"=952.6636881702325, "Y"=3342.7916921165966}, {"X"=952.7474978684022, "Y"=3359.091554695986}, {"X"=954.9294148586805, "Y"=3375.478517435108}, {"X"=960.2101388711521, "Y"=3391.956077999096}, {"X"=971.5896340437512, "Y"=3408.572716688413}, {"X"=974.0768960605492, "Y"=3424.7879517829642}, {"X"=981.6628112449193, "Y"=3441.081700787105}, {"X"=981.3505848148575, "Y"=3457.1486248702304}, {"X"=993.1363215681313, "Y"=3473.3398786074254}, {"X"=994.0218032440225, "Y"=3489.3398859076315}, {"X"=1020.0053964340373, "Y"=3505.2768902312037}, {"X"=1022.0862755609401, "Y"=3521.09097789895}, {"X"=1022.2642158658068, "Y"=3536.908362115882}, {"X"=1025.5385789953302, "Y"=3552.663001800286}, {"X"=1025.91017660836, "Y"=3568.4586087471434}, {"X"=1014.3851121986418, "Y"=3584.6442672599346}, {"X"=975.9825976478487, "Y"=3602.0229001404546}, {"X"=947.6873481122784, "Y"=3619.426113711875}, {"X"=927.497508824365, "Y"=3636.771468735349}, {"X"=928.3870318839645, "Y"=3653.1670610615342}, {"X"=905.4253651296312, "Y"=3671.0775763015645}, {"X"=1015.481200145904, "Y"=3743.8822937417594}, {"X"=1026.9761083045855, "Y"=3758.735488027024}, {"X"=1028.6121158613832, "Y"=3774.518395203543}, {"X"=1030.3449347186652, "Y"=3790.29096691764}, {"X"=1029.195583743087, "Y"=3806.4076587716963}, {"X"=1031.1240604595514, "Y"=3822.1760500878013}, {"X"=-10.842185123417494, "Y"=3975.376392065428}, {"X"=-7.85735733306592, "Y"=3997.523154373408}, {"X"=-13.64461180448643, "Y"=4020.9353314725367}, {"X"=-10.380186862304981, "Y"=4043.0984315132105}, {"X"=-6.979833146683177, "Y"=4065.2410842048967}, {"X"=-1.4697297999809962, "Y"=4087.0407015995165}, {"X"=2.2000808792763564, "Y"=4109.12785355368}, {"X"=6.005346692003968, "Y"=4131.19207218844}, {"X"=10.929770378021203, "Y"=4153.0535099371555}, {"X"=16.96985273450491, "Y"=4174.693236802181}, {"X"=21.177142139041734, "Y"=4196.665595570732}, {"X"=25.51917220141786, "Y"=4218.611725273365}, {"X"=29.995779446655888, "Y"=4240.530799650704}, {"X"=34.606795333023456, "Y"=4262.421993461985}, {"X"=39.35204625837832, "Y"=4284.2844825161355}, {"X"=44.23135356670491, "Y"=4306.117443702798}, {"X"=50.2184105341189, "Y"=4327.69297876029}, {"X"=54.39139747939407, "Y"=4349.6914956217215}, {"X"=60.64276863692294, "Y"=4371.191935682311}, {"X"=66.05492926119678, "Y"=4392.892623444115}, {"X"=71.60014091999074, "Y"=4414.559694303313}, {"X"=76.31174166907931, "Y"=4436.449175396509}, {"X"=78.26458215041703, "Y"=4459.103564097132}, {"X"=80.36291249774058, "Y"=4481.769205199782}, {"X"=86.453191266457, "Y"=4503.346810847743}, {"X"=92.675753086658, "Y"=4524.88664105537}, {"X"=99.03036368240737, "Y"=4546.387884860228}, {"X"=96.90968228848942, "Y"=4570.479904508192}, {"X"=101.63490128460626, "Y"=4592.550518781641}, {"X"=108.40452097556545, "Y"=4613.995516533227}, {"X"=117.20720403105815, "Y"=4634.778983038918}, {"X"=124.23563956341286, "Y"=4656.127635998224}, {"X"=116.24405358750664, "Y"=4682.575792850332}, {"X"=1470.8259571533572, "Y"=4356.529564736725}, {"X"=1476.1216048608221, "Y"=4369.577807134607}, {"X"=1493.49744902776, "Y"=4377.593871188402}, {"X"=1498.9219181053986, "Y"=4390.502607397701}, {"X"=1938.6303433573366, "Y"=4228.317831710194}, {"X"=1943.130492374914, "Y"=4238.4980939056}, {"X"=2064.2835911828975, "Y"=4195.824052250209}, {"X"=2157.596803563967, "Y"=4164.241687122327}, {"X"=2184.342933978691, "Y"=4162.483261240568}, {"X"=2240.815053624293, "Y"=4146.251716860904}, {"X"=2273.6207227573095, "Y"=4140.661387084596}, {"X"=2307.20330673012, "Y"=4134.252875334802}, {"X"=2353.1869782092754, "Y"=4121.213561259799}, {"X"=2382.006623386713, "Y"=4116.211923388506}, {"X"=2411.6065232364003, "Y"=4110.423577842243}, {"X"=2447.295432626557, "Y"=4101.059215349373}, {"X"=2473.9850587374376, "Y"=4095.9583475826716}, {"X"=2498.805913782341, "Y"=4091.4994374293647}, {"X"=2516.504578766092, "Y"=4090.5875651968613}, {"X"=2551.6517061741442, "Y"=4079.8015650482653}, {"X"=2575.2872437016113, "Y"=4074.968492249235}, {"X"=2594.4778607566627, "Y"=4072.3410062991315}, {"X"=2611.865014281955, "Y"=4070.5}, {"X"=2636.9576668055656, "Y"=4063.91973229833}, {"X"=2659.3520795735667, "Y"=4058.5852574114597}, {"X"=2678.2173574415674, "Y"=4055.061041578305}, {"X"=2691.0289338111706, "Y"=4054.9744145738096}, {"X"=2721.660278831192, "Y"=4043.6987531870027}, {"X"=2739.4124804842736, "Y"=4040.041777322615}, {"X"=2750.3361329295954, "Y"=4040.4815565724384}, {"X"=2767.115634515412, "Y"=4037.014556349579}, {"X"=2782.982986635797, "Y"=4033.9093554840906}, {"X"=2807.9514900820814, "Y"=4024.5561532732263}, {"X"=2814.50634246743, "Y"=4027.177118221292}, {"X"=2830.9861725688024, "Y"=4022.9892285885253}, {"X"=2853.1485517299434, "Y"=4014.6473688040373}, {"X"=2857.1403612634576, "Y"=4018.6478160912407}, {"X"=2872.582789543413, "Y"=4014.533965770538}, {"X"=2885.50776424397, "Y"=4011.997895546798}, {"X"=2893.5183185882197, "Y"=4012.847573680118}, {"X"=2899.900941786414, "Y"=4014.8031747070427}, {"X"=2912.6967434174403, "Y"=4011.9211203798964}, {"X"=2931.0186065410116, "Y"=4004.685937198244}, {"X"=2945.2522496038464, "Y"=4000.2813042191124}, {"X"=2954.661095425663, "Y"=3999.3933301945417}, {"X"=2967.182500916552, "Y"=3995.94154177057}, {"X"=2976.503747613994, "Y"=3994.8418164025816}, {"X"=2988.905267857863, "Y"=3991.1407418939402}, {"X"=2993.4815525575614, "Y"=3993.618651300793}, {"X"=3003.4671589723284, "Y"=3991.6071292968145}, {"X"=3015.7083674570613, "Y"=3987.569777714234}, {"X"=3022.5302826587013, "Y"=3987.918769421469}, {"X"=3030.0942129466903, "Y"=3987.552452442963}, {"X"=3046.702190705782, "Y"=3979.2551869622475}, {"X"=3057.1716590001784, "Y"=3976.0476785022497}, {"X"=3067.5806510774983, "Y"=3972.729983069553}, {"X"=3074.953442415055, "Y"=3971.9768133798516}, {"X"=3079.338473615689, "Y"=3973.843407618128}, {"X"=3090.3454777343677, "Y"=3969.5756253620816}, {"X"=3094.698855111437, "Y"=3971.3297709399512}, {"X"=3103.4168856555025, "Y"=3968.92879048734}, {"X"=3107.7491971523373, "Y"=3970.584898924553}, {"X"=3123.58038741206, "Y"=3961.0784670113726}, {"X"=3127.132781099316, "Y"=3963.2932044495506}, {"X"=3141.3442900960695, "Y"=3954.9186078547696}, {"X"=3145.5555703671926, "Y"=3956.307199565942}, {"X"=3151.8704643852734, "Y"=3955.5226880296186}, {"X"=3156.0677567657553, "Y"=3956.8294686390223}, {"X"=3159.5716639723732, "Y"=3958.823365603732}, {"X"=3175.4683402686765, "Y"=3947.7296839453106}, {"X"=3178.2235496518883, "Y"=3950.3261328545645}, {"X"=3180.994638680067, "Y"=3952.9056272394423}, {"X"=3195.249435679037, "Y"=3942.9187066289505}, {"X"=3197.974753086856, "Y"=3945.3938715838212}, {"X"=3201.380681173798, "Y"=3947.1058472649793}, {"X"=3206.7751036892987, "Y"=3946.541354099974}, {"X"=3212.803756375196, "Y"=3945.173077491038}, {"X"=3218.8006896511197, "Y"=3943.7477727150167}, {"X"=3224.1184753772477, "Y"=3943.0283054696115}, {"X"=3228.7707174038055, "Y"=3943.026883770178}, {"X"=3236.596467994627, "Y"=3939.1330924970466}, {"X"=3243.09464444919, "Y"=3936.7087899036956}, {"X"=3247.0370537459103, "Y"=3937.33414978896}, {"X"=3255.336482079424, "Y"=3932.453534399492}, {"X"=3258.6149065322234, "Y"=3933.7743860095907}, {"X"=3264.351012075589, "Y"=3931.9129043051607}, {"X"=3269.4425440482646, "Y"=3930.7908637781406}, {"X"=3272.6959317916744, "Y"=3932.0139429859637}, {"X"=3277.1498206927595, "Y"=3931.6118183290196}, {"X"=3284.5566606113143, "Y"=3927.1492709057507}, {"X"=3290.7181866922274, "Y"=3924.2284289826134}, {"X"=3293.3270255400894, "Y"=3926.118160532863}, {"X"=3297.105706031337, "Y"=3926.3614038362584}, {"X"=3304.8947253046604, "Y"=3920.8430548874344}, {"X"=3308.6207253100038, "Y"=3921.001328122765}, {"X"=3311.2094260290082, "Y"=3922.7812725103904}, {"X"=3314.926933145405, "Y"=3922.8869193461956}, {"X"=3318.0809533830084, "Y"=3923.7955298897887}, {"X"=3324.527865814621, "Y"=3919.6654659217893}, {"X"=3329.8261174974987, "Y"=3917.1511395328134}, {"X"=3334.0061420335082, "Y"=3916.2730684587964}, {"X"=3338.165158372983, "Y"=3915.359501769437}, {"X"=3341.2467531813195, "Y"=3916.109068948024}, {"X"=3349.556141722818, "Y"=3908.312225938973}, {"X"=3352.0662129768757, "Y"=3909.8412342021875}, {"X"=3356.12266085134, "Y"=3908.7784772340265}, {"X"=3358.635469356694, "Y"=3910.2671853162724}, {"X"=3361.659135341594, "Y"=3910.875446131651}, {"X"=3366.6669726322425, "Y"=3907.989826269476}, {"X"=3370.1569787062945, "Y"=3907.671663919117}, {"X"=3375.5773121030506, "Y"=3903.8297378315624}, {"X"=3379.9809532133554, "Y"=3901.6909496753647}, {"X"=3381.0248231909495, "Y"=3905.6733562134013}, {"X"=3384.9268861109003, "Y"=3904.360675241852}, {"X"=3387.4120452614275, "Y"=3905.672727084371}, {"X"=3391.740097239402, "Y"=3903.415186751994}, {"X"=3396.9388950941193, "Y"=3899.337185439076}, {"X"=3399.3930045680063, "Y"=3900.5756275458457}, {"X"=3402.2969554721067, "Y"=3900.902115465112}, {"X"=3404.7605663121444, "Y"=3902.107651672093}, {"X"=3407.231527806511, "Y"=3903.2980487532614}, {"X"=3410.1354521890526, "Y"=3903.5684000074143}, {"X"=3415.9764364638286, "Y"=3897.4661344862584}, {"X"=3419.2478453327217, "Y"=3896.7677640423126}, {"X"=3421.685769173619, "Y"=3897.8693693724063}, {"X"=3424.1304064445235, "Y"=3898.9559951456195}, {"X"=3428.570407478858, "Y"=3895.4401279688686}, {"X"=3431.000009603355, "Y"=3896.484556125373}, {"X"=3434.595352849846, "Y"=3894.747137673135}, {"X"=3437.0205894479313, "Y"=3895.754610505172}, {"X"=3440.2021866047417, "Y"=3894.893224598871}, {"X"=3442.997631366253, "Y"=3894.937028199931}, {"X"=3445.7875834697406, "Y"=3894.9614292407523}, {"X"=3447.855938217865, "Y"=3896.8339507456913}, {"X"=3453.1117300168457, "Y"=3890.272771457805}, {"X"=3455.509163854388, "Y"=3891.166714164104}, {"X"=3457.912037690245, "Y"=3892.0459296647036}, {"X"=3460.9901878630535, "Y"=3891.0259225801415}, {"X"=3465.367148692672, "Y"=3886.2058976101466}, {"X"=3467.7393979566095, "Y"=3887.0247190388745}, {"X"=3470.7517532769834, "Y"=3885.9324950286336}, {"X"=3473.433962618886, "Y"=3885.7681145217193}, {"X"=3475.497470820703, "Y"=3887.489509829567}, {"X"=3479.0776275398593, "Y"=3884.430461642429}, {"X"=3482.0271182627307, "Y"=3883.2537007970104}, {"X"=3483.804285900354, "Y"=3885.8854182589353}, {"X"=3486.7391138662306, "Y"=3884.672551233115}, {"X"=3490.4843260336584, "Y"=3880.555274770562}, {"X"=3492.821430903891, "Y"=3881.2200864677916}, {"X"=3494.6330890219583, "Y"=3883.7991845626375}, {"X"=3497.507658139402, "Y"=3882.506627210471}, {"X"=3499.8566040708733, "Y"=3883.1283078183887}, {"X"=3502.9501588268386, "Y"=3880.828476257047}, {"X"=3505.2887053640984, "Y"=3881.4167938992614}, {"X"=3507.6308177280707, "Y"=3881.9907514147626}, {"X"=3510.434543069118, "Y"=3880.603506190842}, {"X"=3513.2177495607757, "Y"=3879.196309328959}, {"X"=3516.631613886397, "Y"=3874.8409158520626}, {"X"=3518.9331638941576, "Y"=3875.3453983783315}, {"X"=3521.6479859911105, "Y"=3873.8782715012344}, {"X"=3524.1426355863878, "Y"=3873.3720132310673}, {"X"=3526.241947276591, "Y"=3874.81161889468}, {"X"=3528.54313660979, "Y"=3875.257134075334}, {"X"=3530.847016253508, "Y"=3875.6885210369855}, {"X"=3532.2785452725334, "Y"=3881.0286138462516}, {"X"=3534.6177677323685, "Y"=3881.4369721247554}, {"X"=3537.448138216478, "Y"=3878.8710395205935}, {"X"=3540.244540164776, "Y"=3876.284845588925}, {"X"=3542.554505452179, "Y"=3876.644414741751}, {"X"=3545.879582520246, "Y"=3870.0634815971675}, {"X"=3548.2899011305954, "Y"=3869.3982480669288}, {"X"=3550.5574595983317, "Y"=3869.7085814511606}, {"X"=3552.953349041593, "Y"=3869.013025018898}, {"X"=3555.459217026101, "Y"=3867.3092956243718}, {"X"=3557.713822962267, "Y"=3867.5756782371946}, {"X"=3560.1863992142376, "Y"=3865.839961174927}, {"X"=3562.4319004958415, "Y"=3866.0773660029336}, {"X"=3564.486853239697, "Y"=3868.291754465371}, {"X"=3566.657445372384, "Y"=3869.498679362869}, {"X"=3568.9252743111374, "Y"=3869.696309723754}, {"X"=3571.1942731957497, "Y"=3869.880021227531}, {"X"=3573.4643565996953, "Y"=3870.049806957566}, {"X"=3575.9970515725377, "Y"=3866.2142248285672}, {"X"=3578.4223891140427, "Y"=3863.359885937419}, {"X"=3580.7586355337407, "Y"=3861.4882707550505}, {"X"=3582.9770480783645, "Y"=3861.5995286333678}, {"X"=3585.196101527507, "Y"=3861.697172493809}, {"X"=3587.346185883872, "Y"=3863.779989812956}, {"X"=3589.5785361435096, "Y"=3863.850784101241}, {"X"=3591.811278765371, "Y"=3863.9078796131535}, {"X"=3594.044329687959, "Y"=3863.9512741990807}, {"X"=3596.2776048381675, "Y"=3863.9809662252396}, {"X"=3598.5232919465293, "Y"=3860.9969796734104}, {"X"=3600.734264958528, "Y"=3858.999249100845}, {"X"=3602.9124856990015, "Y"=3855.988086074595}, {"X"=3605.1110493698097, "Y"=3856.963411534487}, {"X"=3607.301239472894, "Y"=3856.9253309897736}, {"X"=3609.491154688439, "Y"=3856.8738124080837}, {"X"=3611.680712567374, "Y"=3856.8088577290628}, {"X"=3613.869830674083, "Y"=3856.730469398217}, {"X"=3616.0584265895063, "Y"=3856.6386503668236}, {"X"=3618.144197085594, "Y"=3854.5360180744956}, {"X"=3620.262010319799, "Y"=3853.4196527328386}, {"X"=3622.4301711150943, "Y"=3853.2886743496706}, {"X"=3624.5974874271237, "Y"=3853.1443948475926}, {"X"=3626.7638776576546, "Y"=3852.9868196586467}, {"X"=3628.847539169185, "Y"=3851.8192994761407}, {"X"=3631.0057187613443, "Y"=3851.6356714044987}, {"X"=3633.068785592103, "Y"=3850.4432270988605}, {"X"=3635.3184946920105, "Y"=3851.2287060202943}, {"X"=3637.3667730516813, "Y"=3850.01103449992}, {"X"=3639.513696966361, "Y"=3849.775167431953}, {"X"=3641.6591332126836, "Y"=3849.5261315266252}, {"X"=3643.803001016186, "Y"=3849.263936159999}, {"X"=3645.9452196614584, "Y"=3848.988591203581}, {"X"=3648.358922747992, "Y"=3850.681357632044}, {"X"=3650.5097527639764, "Y"=3850.3780313828506}, {"X"=3652.658681116318, "Y"=3850.06151359881}, {"X"=3654.805626899078, "Y"=3849.731816196638}, {"X"=3656.9505092809613, "Y"=3849.3889515892556}, {"X"=3659.093247508359, "Y"=3849.0329326853207}, {"X"=3661.233760908388, "Y"=3848.663772888745}, {"X"=3663.371968891928, "Y"=3848.2814860981853}, {"X"=3665.507790956657, "Y"=3847.8860867065237}, {"X"=3667.6411466900818, "Y"=3847.4775896003234}, {"X"=3669.771955772565, "Y"=3847.05601015927}, {"X"=3672.3063534491635, "Y"=3848.579677047995}, {"X"=3674.6529488935626, "Y"=3849.107343408149}, {"X"=3676.7936259622215, "Y"=3848.642709677937}, {"X"=3678.931411794267, "Y"=3848.1649497467597}, {"X"=3681.9745309554087, "Y"=3851.5695895191175}, {"X"=3682.265797573908, "Y"=3843.2802623943426}, {"X"=3684.3705770359, "Y"=3842.7690267959306}, {"X"=3685.982252627952, "Y"=3840.3058216266995}, {"X"=3689.072343340926, "Y"=3843.6438820228814}, {"X"=3690.408697130985, "Y"=3840.191515889326}, {"X"=3692.7571392126815, "Y"=3840.5952335618913}, {"X"=3694.845246150937, "Y"=3840.019674846277}, {"X"=3696.929782219281, "Y"=3839.4313145820856}, {"X"=3699.01066893611, "Y"=3838.830174920747}, {"X"=3701.0878279572144, "Y"=3838.2162784948305}, {"X"=3702.868939772559, "Y"=3836.6333038041093}, {"X"=3704.336338764959, "Y"=3834.086707926436}, {"X"=3706.9922024064654, "Y"=3835.3455958026198}, {"X"=3707.4988553411154, "Y"=3829.928774283708}, {"X"=3709.5212366069845, "Y"=3829.262962891481}, {"X"=3712.1823733908036, "Y"=3830.478615193792}, {"X"=3714.8625275878517, "Y"=3831.6739359011044}, {"X"=3716.8954783450504, "Y"=3830.9629090132034}, {"X"=3718.9240280535587, "Y"=3830.239421558839}, {"X"=3721.9818447869743, "Y"=3832.3197700143137}, {"X"=3725.069629579242, "Y"=3834.3749209449047}, {"X"=3726.0507345592364, "Y"=3830.79784206835}, {"X"=3728.078099090901, "Y"=3830.01818212526}, {"X"=3730.1006415545253, "Y"=3829.22609718414}, {"X"=3731.7450703059103, "Y"=3827.493872385562}, {"X"=3732.994252855881, "Y"=3824.8284604330506}, {"X"=3734.984859240635, "Y"=3824.006308234556}, {"X"=3737.750841547497, "Y"=3825.0133930362813}, {"X"=3741.3259774571916, "Y"=3827.8352758562896}, {"X"=3743.3348764721827, "Y"=3826.9619445542617}, {"X"=3745.338379010088, "Y"=3826.0763033198214}, {"X"=3747.3364096401688, "Y"=3825.17838549686}, {"X"=3749.747181353774, "Y"=3825.176539246914}, {"X"=3751.739608140834, "Y"=3824.2515864591355}, {"X"=3753.7263220174113, "Y"=3823.314425782394}, {"X"=3755.707248184851, "Y"=3822.3650925002603}, {"X"=3758.563218833701, "Y"=3823.19917331747}, {"X"=3760.989300513128, "Y"=3823.1152195739064}, {"X"=3762.5174303442213, "Y"=3821.229022403504}, {"X"=3764.9422991025817, "Y"=3821.11530322729}, {"X"=3766.909520570095, "Y"=3820.0971914013944}, {"X"=3770.273813595049, "Y"=3821.718554646446}, {"X"=3772.244636179431, "Y"=3820.6677179065823}, {"X"=3774.208973850614, "Y"=3819.604808208381}, {"X"=3775.1988034619967, "Y"=3816.779701473255}, {"X"=3776.1605593274253, "Y"=3813.95454661057}, {"X"=3778.083632037759, "Y"=3812.8677356331905}, {"X"=3781.0, "Y"=3813.5011961699665}]}]
  in  "stop":bool
  # "max. distance (mm)\nto the furthest outlier"
  # "shortest allowable line\n(points)"
  # "max. angle deviation\n(degrees) from a\nhorisontal or vertical"
  # "max. adjacent angle\n(degrees) deviation\nfor merge"
  # "minimum distance (mm)\nto merge corners"
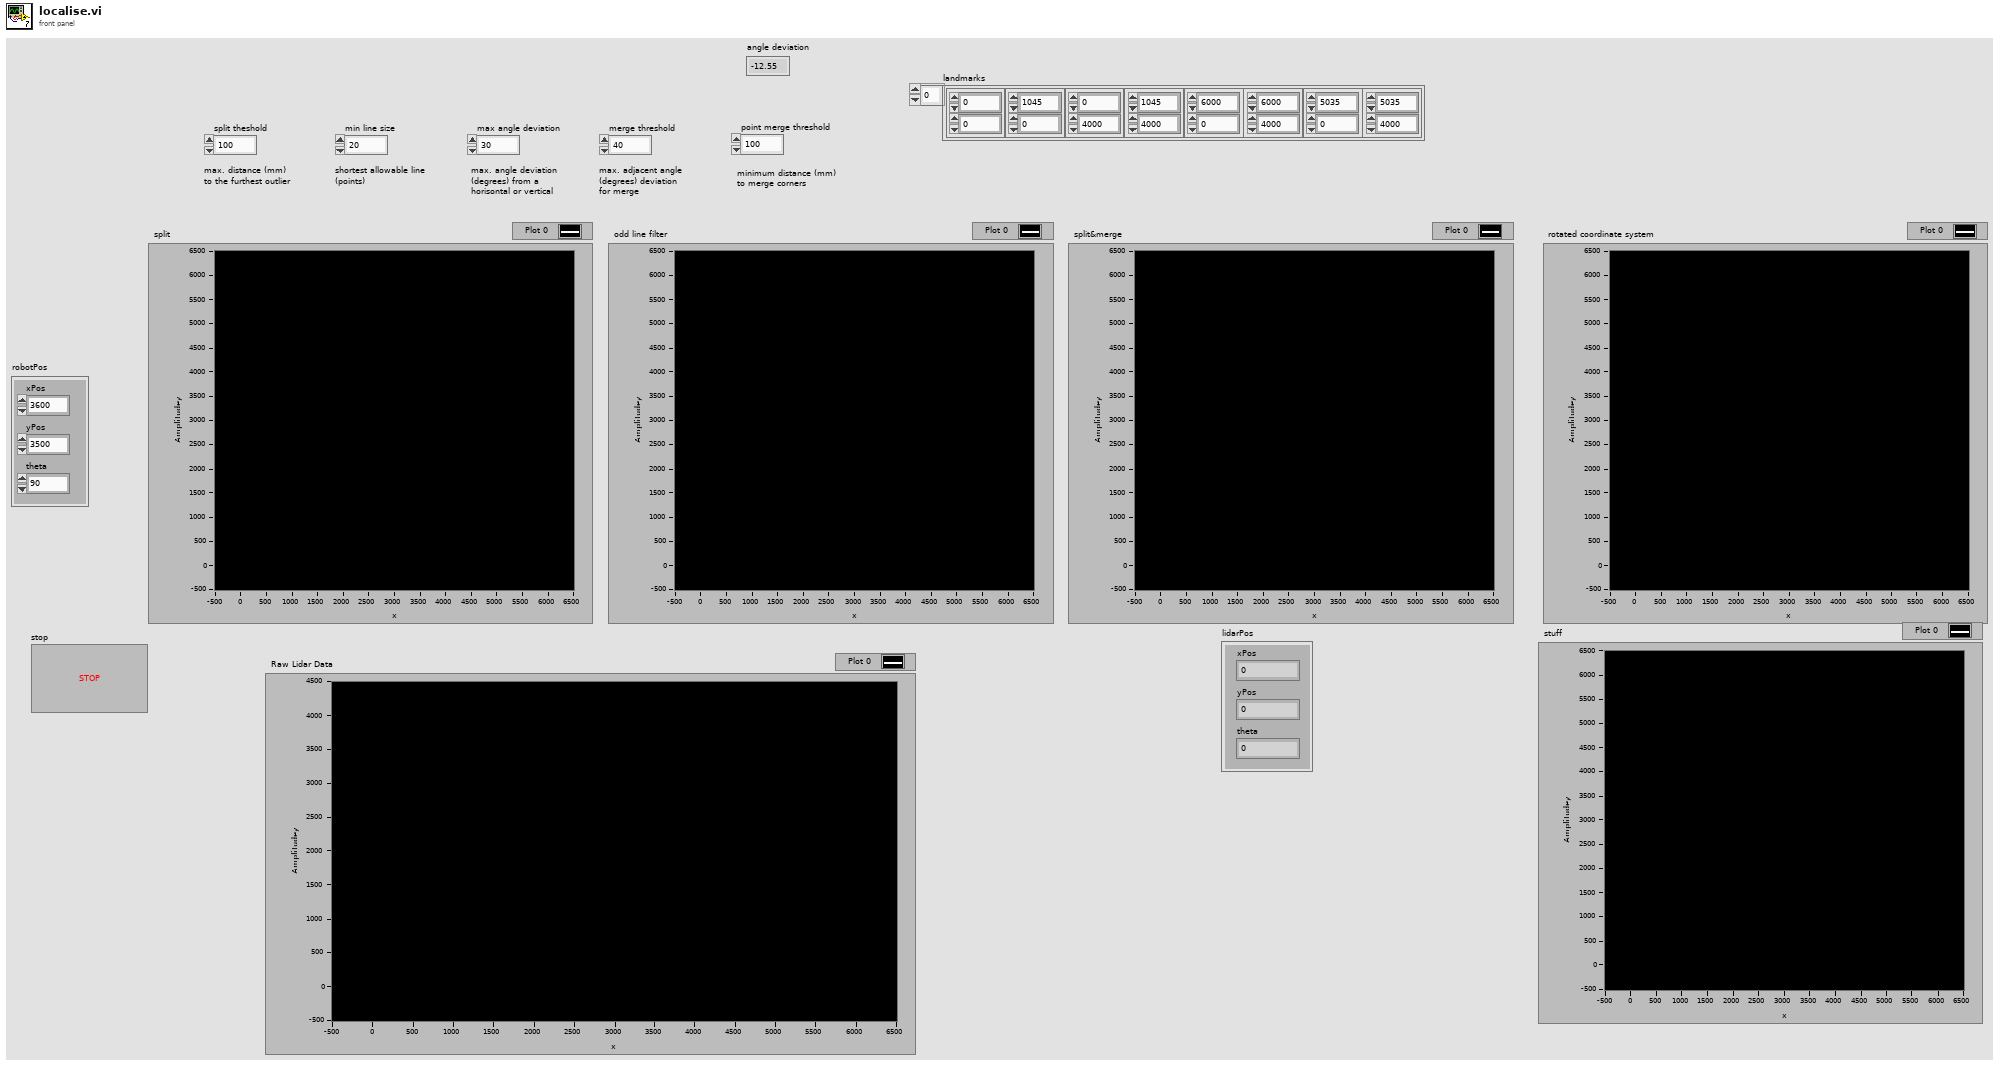
[diagram p1: front panel]
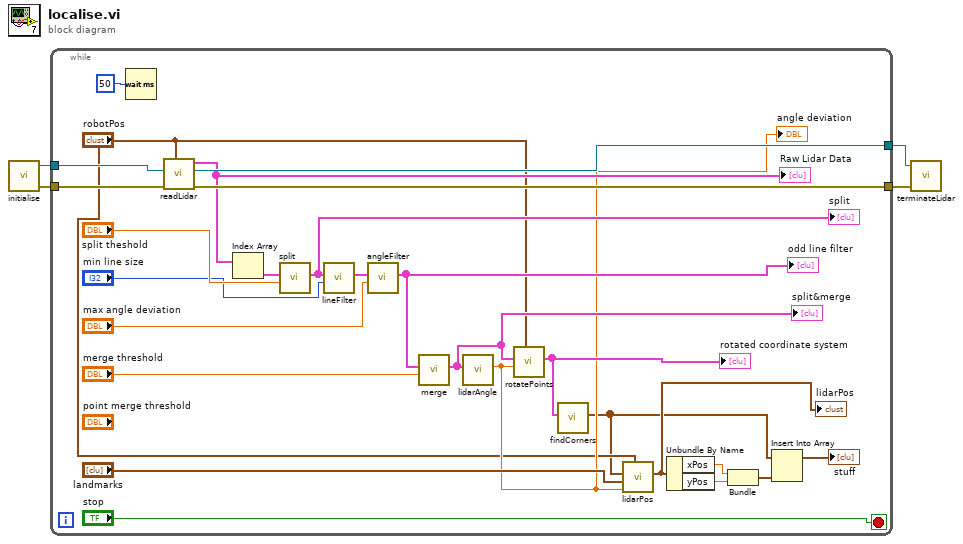
[diagram p0: block diagram]
diagram:
  n1 = call "initialise.vi"() -> ("error out"=w3:errorcluster, "VISA resource name out"=w4:refnum<visa-resource-name>)  [unwired: 4 in]
  n2 = while {
    tunnel: w4 -> [w30]
    tunnel: w3 -> [w29]
    tunnel: [w28] -> w2
    tunnel: [w27] -> w1
    stop <- "stop" stop-if-true
    n3 = Wait (ms)(milliseconds to wait=u32 50) -> ()  [unwired: 1 out]
    n4 = call "readLidar.vi"("robotPos"="robotPos", "error in"=w29, "VISA resource name in"=w30) -> ("error out"=w27:errorcluster, "VISA resource name out"=w28:refnum<visa-resource-name>, "line out"=w24:cluster{"Line":cluster{"X":dbl, "Y":dbl}[]}[])  [unwired: 3 in, 1 out]
    "Raw Lidar Data" <- w24
    n5 = Index Array(array=w24) -> (element=w23:cluster{"Line":cluster{"X":dbl, "Y":dbl}[]})  [unwired: 1 in]
    n6 = call "split.vi"("Threshold"="split theshold", "points in"=w23) -> ("line out"=w19:cluster{"Line":cluster{"X":dbl, "Y":dbl}[]}[])  [unwired: 9 in]
    "split" <- w19
    n7 = call "lineFilter.vi"("min line size"="min line size", "Input"=w19) -> ("Output"=w18:cluster{"Line":cluster{"X":dbl, "Y":dbl}[]}[])  [unwired: 9 in]
    n8 = call "angleFilter.vi"("max angle deviation"="max angle deviation", "Input"=w18) -> ("Output"=w16:cluster{"Line":cluster{"X":dbl, "Y":dbl}[]}[])  [unwired: 9 in]
    "odd line filter" <- w16
    n9 = call "merge.vi"("Merge Threshold"="merge threshold", "Input"=w16) -> ("Output"=w15:cluster{"Line":cluster{"X":dbl, "Y":dbl}[]}[])  [unwired: 9 in]
    "split&merge" <- w15
    n10 = call "lidarAngle.vi"("Input"=w15) -> ("average"=w12:dbl)  [unwired: 10 in]
    "angle deviation" <- w12
    n11 = call "rotatePoints.vi"("robotPos"="robotPos", "angle deviation"=w12, "Input"=w15) -> ("Output"=w14:cluster{"Line":cluster{"X":dbl, "Y":dbl}[]}[])  [unwired: 8 in]
    "rotated coordinate system" <- w14
    n12 = call "findCorners.vi"("Input"=w14) -> ("corners"=w7:cluster{dbl, dbl}[])  [unwired: 10 in]
    n13 = call "lidarPos.vi"("robotPos"="robotPos", "angle deviation"=w12, "landmarks"="landmarks", "corners"=w7) -> ("lidarPos"=w10:cluster{"xPos":dbl, "yPos":dbl, "theta":dbl})  [unwired: 7 in]
    "lidarPos" <- w10
    n14 = Unbundle By Name(w10) -> ("xPos"=w9:dbl, "yPos"=w8:dbl)
    n15 = Bundle("xPos"=w9, "yPos"=w8) -> (w6:cluster{"xPos":dbl, "yPos":dbl})  [unwired: 1 in]
    n16 = Insert Into Array(array=w7, new element=w6) -> (→"stuff":cluster{dbl, dbl}[])  [unwired: 1 in]
  }
  n17 = call "terminateLidar.vi"("error in"=w1, "VISA resource name"=w2) -> ()  [unwired: 3 in, 1 out]
